vi "Argos_K_4.2 (SUPTNIK Customized Edition).vi"(0 "PID 1 COM":refnum<visa-resource-name>="COM1", 1 "Setpoint\n START":bool, 2 "Write to File":bool, 3 "SP 1 input (°C)":dbl=20.0 min=0.0 max=1300.0, 4 "Intervall (s)":u32=1 max=600, 5 "Write/\nRead":bool=TRUE, 6 "Delay (ms)":u32=500 min=100 max=600000, 7 "Auto Tune":bool, 9 "Standby":bool, 11 "Reset\nSTOPP":bool, 12 "ON":bool=TRUE caption="OFF", 13 "Get Values":bool, 15 "File Path":path) -> (8 "(°C)":dbl format="%#.3f", 14 "SP 1 is (°C)":dbl)   [LabVIEW 2013]
doc: "1. Verwendung\n\nDas Programm dient der Steuerung und Abfrage des Thermocontrollers I3252 und dem Auslesen von zwei VC 840 Messgeräten und einem Druckmessgerät Pfeiffer Single Gauge. \nDie Messgeräte werden Standardmäßig ausgelesen und erst nach Betätigung des Schalters \"Write to File\" in einer Textdatei abgespeichert. Das Eingabefeld \"Intervall\" legt den Abstand der Messpunkte fest.\nDer Setpoint für den Thermocontroller wird erst nach Betätigung des Tasters \"Setpoint START\" übernommen und angesteuert. Er wird ind den EEPROM des Gerätes geschrieben. Die Regelung kann mit Hilfe des Schalters \"Standby\" unterbrochen werden. Durch den Taster \"Reset STOPP\" kann der Setpoint aus dem EEPROM gelöscht werden.\nDie Eingabeflächen \"Constant\" und \"Thickness\" dienen der Berechnung des spezifischen Widerstands.\nDie Eingabeflächen \"User\" und \"Sample\" werden in den Header der Textdatei übernommen.\nDer Indikator \"File Path\" zeigt den aktuellen Speicherort der Textdatei an. Dieser wird nach ausschalten des Schalters \"Write to File\" gelöscht. Bei erneuten Schreiben muss ein neuer Speicherort gewählt werden. Bei Wahl desselben Speicherorts werden sämtliche bereits gespeicherte Daten gelöscht.\n\n\n2. Erläuterungen zum Blockdiagramm\n2.1 äußere Sequenz\nDie äußerte Sequenz besteht aus fünf Frames. Der erste dient der Initialisierung der Ports. Der zweite dient als Verzögerung um dem Programm genug Zeit zu geben die Ports zu öffnen. Jedoch senden die beiden VC 840 bereits Informationen an den Computer die in einem Puffer zwischengespeichert werden. Im dritten Frame wird dieser Puffer geleert. Somit kommt es zu keinem Framing Error. Desweiteren wird in diesem Frame die Startzeit der Messungen genommen. Im vierten Frame wird die eigentliche Messung und Verarbeitung der Daten durchgeführt. Die while-Schleife wird nur durch Auftreten eines Fehlers oder durch Betätigung des Stopbuttons auf dem Front Panel in der oberen linken Ecke unterbrochen. Im fünften und letzten Frame werden die Ports wieder geschlossen und beim Auftreten eines Fehlers wird das Programm automatisch gestoppt. Falls kein Fehler auftritt wird die Sequenz von vorne abgearbeitet.\n\n2.2 while-Schleife und innere Sequenz\n2.2.1 \"Event Structure\"\n2.2.1.1 Allgemein\nDer erste Frame beinhaltet ein \"Event Structure\". Dieser reagiert auf insgesamt elf verschiedene Ereignisse. Falls keines dieser Ereignisse auftreten sollte, warte die Struktur eine Millisekunde bevor die \"Event Structure\" verlassen wird. Die übrigen Ereignisse treten ein, wenn der entsprechende Kontroller eine Werteänderung erfährt.\n\n2.2.1.2 Event: Setpoint\nDieser Case besteht von außen nach innen aus einer Stacked Sequence, einer for-Loop und einer Flat Sequence die wiederum zwei \"Case Structures\" enthält. Als erstes wird bei dem Schalter \"Setpoint START\" der Blinkmodus aktiviert und bei dem Schalter \"Read Temperature\" deaktiviert. Danach folgt das eigentliche setzen des Temperatursollwerts. In der ersten Iteration wird dem Controller I3252 ein Schreibbefehl gesendet. Theoretisch kann der Setpoint in den RAM oder in den EEPROM geschrieben werden. Diese Auswahl erfolgt mit Hilfe des Schalters \"RAM\". Da das Schreiben in den RAM -Speicher aber aus diversen Gründen nicht erwünscht ist, wurde es nicht implementiert. Eine nachträgliche Implementierung ist aber leicht möglich, in dem die untere String-Konstante \"*P012\" durch \"*W012\" ersetzt wird. An diesem Befehl wird eine fünfstellige Hexadezimalzahl angehängt, die den Sollwert wiedergibt. Der Sollwert wird vorher mit zehn multipliziert, da das Komma standardmäßig nach der ersten Ziffer festgesetzt wurde (Bsp.: 800 wird gesendet um 80 einzustellen). Dieser Befehlsstrang wird an das Gerät mittels des SubVIs \"Comm_Interface\", auf welches später noch näher eingegangen wird, weitergegeben. Der durch das Gerät zurückgegebene String wird nicht verarbeitet.\nDie zweite Iteration dient dem Auslesen des eingestellten Sollwertes. Wahlweise kann der RAM- oder der EEPROM-Speicher ausgelesen werden. Die eigentliche Verarbeitung des Ausgabestrings erfolgt durch das SubVI \"Edit Setpoint\".\nDie Implementierung zur Einstellung des zweiten Setpoints erfolgt durch kopieren der ersten beiden Fälle und ersetzen der \"1\" im Befehf durch eine \"2\" (Bsp.: \"*P012\" zu \"*P022\"). Es darf aber nicht vergessen werden, dass dann ebenfalls die Anzahl der Iterationen angepasst werden muss.\nAls letztes wird der Blinkmodus des Schalters \"Setpoint START\" wieder deaktiviert.\n\n2.2.1.3 Event: Standby\nDieses Ereignis aktiviert bzw. deaktiviert als erstes den Blinckmodus des entsprechenden Schalters und sendet danach den Befehl zum aktivieren (\"*D03\") oder zum deaktivieren (\"*E03\") des Standbymodus an den Thermocontroller.\n\n2.2.1.4 Event: Set Command \nDer in das Feld \"Command shall be\" eingegebene Befehl wird an den Thermocontroller übermittlet. Die korrekte Form des Befehls ist im \"Communication Manuel\" nachzuschlagen. Das \"*\"-Zeichen wurde allerdings schon implementiert und muss somit nicht mit eingegeben werden.\n\n2.2.1.5 Event: Reset\nIn der ersten Iteration wird der Reset-Befehl an den Thermocontroller gesendet. In Folge wird der gesamte EEPROM-Speicher gelöscht. Deshalb wird in der zweiten Iteration der Setpoint aktualisiert. Dieser Befehl hat keinen Einfluss auf den RAM-Speicher. Die anschließende Wartezeit ist auf vier Sekunden festgesetzt und wurde empirisch ermittelt. Diese Zeit benötigt das Gerät um den Reset durchzuführen und für die Kommunikation wieder zur Verfügung zu stehen.\n\n2.2.1.6 Event: Auto Tune\nEs ist festgeschrieben, dass der Setpoint für die \"Auto Tune\"-Funktion wenigstens 20°C über der aktuellen Temperatur liegt. Deshalb wird zunächst der aktuelle Temperaturwert ausgelesen. Im zweiten Schritt werden zu diesem Wert zwanzig addiert und der Setpoint wird in den RAM-Speicher geschrieben. Das Schreiben in diesen Speicher ist nötig, da die \"Auto Tune\"-Funktion\" erst nach einem Reset startet. Im dritten Schritt wird der eigentliche Befehl für den \"Auto Tune\" gesendet (siehe dazu \"Communication Manuel\" S.27). Als vierte und letzte Iteration der for-Schleife folgt der bereits erwähnte Reset-Befehl. Der Temperatursollwert, der im RAM-Speicher eingetragen ist, muss zum Schluss wieder auf 0°C gesetzt werden. Die Zeit für die Ausführung des \"Auto Tune\"-Befehls wurde empirisch ermittelt und 45 s festgesetzt.\n\n2.2.1.7 Event: Write LOW/HI\nDieses Ereignis setzt die am Analogausgang anliegende Spannung fest. Normalerweise beträgt dieser Spannungswert 0-10 V. Das angeschlossene Netzteil verträgt aber maximal nur 2,3 V. Aus diesem Grund wird der \"%HIGH\" auf 23 gesetzt. Somit beträgt die maximal anliegende Spannung nur noch 23% von der maximal möglichen, d.h 2,3V. Ein niedrigerer Wert ist jederzeit möglich, genauso wie ein höherer für den Parameter \"%LOW\". Diese werden zunächst nacheinander in den RAM-Speicher geschrieben und anschließend wieder ausgelesen.\n\n2.2.1.8 Event: Set PID\nDie Werte für den PID-Regler können sowohl mit Hilfe der \"Auto Tune\"-Funktion, als auch manuell eingestellt werden. Es wird wiederum zwischen dem Schreiben in den RAM- und dem EEPROM-Speicher unterschieden. Zunächst werden die Werte für \"P\", \"I\" und \"D\", in dieser Reihenfolge, gesetzt und danach die aktuellen Werte ausgelesen.\n\n2.2.1.9 Event: Get Values\nDieses Ereignis hat zur Folge, dass die Werte für \"P\", \"I\", \"D\", \"%LOW\", \"%HIGH\" und des Setpoints wahlweise aus dem RAM- oder EEPROM-Speicher gelesen werden. Die aktuellen Werte werden nicht nur in die entsprechenden Anzeigefelder übernommen, sondern auch in die entsprechenden Eingabefelder, mit Ausnahme des Temperatursollwerts. \n\n2.2.1.10 Event: RAM\nPrinzipiell kann zwischen dem Schreiben in den RAM- oder EEPROM-Speicher des Thermocontrollers gewählt werden. Die entsprechende Schalterposition auf dem Frontpanel zeigt den aktuell verwendeten Speicher an. Die Anzeigewerte werden bei jedem Umschalten aktualisiert und sind im entsprechenden Speicher eingetragen. Die Implementierung ist identisch mit der des Ereignisses \"Get Values\". Es gilt zu beachten, dass die Werte für \"%LOW\" und \"%HIGH\" nur in den RAM-Speicher geschrieben werden können und somit auch nur aus diesem ausgelesen werden können.\n\n2.2.1.11 Event: Set Gauge to Zero\nMit Hilfe der SubVIs \"Get Pressure\" und \"Offset Display\" werden die Werte für den alten und den neuen Offset und der durch den zweiten Drucksensor ermittelt Druck ermittelt. \n\n2.2.1.12 Event: Write to File\nSollte der Schalter \"Write to File\" aktiviert werden, d.h. Schalterposition oben, so wird zunächst durch das SubVI \"Header\" ein Header für die unter \"File Path\" definierte Datei angelegt. Alle Werte, die bereits in der entsprechenden Datei stehen, werden dabei gelöscht.\n\n2.2.2 \"Timed Structures\"\nIm dritten Frame der inneren Sequenz werden die Werte für Zeitpunkt, Temperatur, Spannung, Strom und Druck ermittelt. Damit die Werte zum gleichen Zeitpunkt aufgenommen werden, werden \"Timed Sequences\" eingesetzt. Mit dem entsprechenden Schalter auf dem Front Panel unter dem Tab \"Settings\" kann gewählt werden, ob das entsprechende Gerät ausgelesen werden soll oder nicht. Die einzelnen Sequenzen werden parallel abgearbeitet, womit die Prozesszeit von diesem Frame durch der zeitintensivsten Sequenz abhängt. Dies ist in aller Regel das Auslesen der Temperatur, da ein \"Delay\" von 500 ms oder größer benötigt wird, um den Controller ordentlich ansprechen zu können.\nDie Systemzeit wird durch das SubVI \"System Time in Seconds\" in Sekunden umgerechnet und der in dem Parameter \"Starttime\" gespeicherte Wert wird abgezogen. Somit werden die Sekunden seit dem Start des Programms gezählt.\n\n2.2.3 restlichen Frames\nIm zweiten Frame wird das Intervall zwischen den einzelnen Messwerten festgelegt. Dabei wird der Wert des Parameters \"Delay\" abgezogen. Dieser Wert beträgt im Normalfall 500 ms und ist somit nicht vernachlääsigbar.\nDer Vierte Frame beinhaltet die Umrechnung des Temperatur-Strings in einen Temperaturwert durch das SubVI \"Edit Tmperature\", die Berechnung des spezifischen Widerstands durch das SubVI \"Resistivity Calculation\" und die Überprüfung des Druckwerts. Auch werden die neu gewonnen Werte in das entsprechende Shift-Register übernommen. Falls der Druckwert einen in dem Parameter \"Pressure Limit (mbar)\" festgelegten Grenzwert überschreiten sollte, wird der Thermocontroller automatisch in den Standby-Modus versetzt. Des Weiteren wird der Schalter \"Standby\" solange gesperrt, wie der Druck oberhalb des Grenzwertes liegt. Wenn der Druck wieder unter den Grenzwert gesunken ist, wird der Standby-Befehl nicht automatisch aufgehoben, sondern muss vom Benutzer durch Betätigung des entsprechenden Schalters gegeben werden.\nIm fünften Frame werden die Diagramme erstellt. Dabei wird jedes Mal von neuem das gesamte Shift-Register als Graph dargestellt. Weiterhin werden die Messwerte in ein 1D-Array geschrieben.\nDer sechste und letzte Frame beinhaltet den eigentlich Schreibvorgang der Messwerte in eine Textdatei und die Überprüfung ob ein Fehler vorliegt.\n\n2.3 SubVIs\n2.3.1 Allgemein\nDie SubVIs für die Messgeräte VC840 und das Druckmessgerät wurden aus anderen Quellen übernommen. \n\n2.3.2 \"Header\"\nIn den Header wird zunächst das aktuelle Datum und die aktuelle Zeit übernommen. Die ausgewählte Datei wird dabei überschrieben. Danach wird der Name des Benutzers und der Probe übernommen. Zum Schluss werden die Einheiten in einer Reihe, durch einen Tabulator getrennt, in den Header geschrieben.\n\n2.3.3 \"I3252 Comm Interface\"\nDieses VI stellt die Kommunikation mit dem Thermocontroller her und gibt den Ausgabe-String zurück.\n\n2.3.4 \"I3252 Edit Setpoint\"\nIm Ausgabe-String vom Thermocontroller ist an der vierten Stelle die Stelle des Dezimalpunktes verschlüsselt. Dieses Hexadezimalzahl wird herausgefiltert und an ein \"ENUM Controller\" übergeben. Dieser weist der Hexadezimalzahl eine Nummer zu, mit welcher ein Wert aus einem Array entnommen wird. Dieser Wert dient als Quotient. Der tatsächliche Wert kann somit errechnet werden.\n\n2.3.5 \"I3252 Edit Temperature\"\nDer Temperatur-String, der vom Thermocontroller zurückgegeben wird, wird in eine Dezimalzahl umgewandelt. Manchmal kommt es aus zu Dropouts, die durch dieses Programm herausgefiltert werden. Der letzte Wert wird dabei in einer \"Feedback Node\" gehalten unter der Annahme, dass sich der Temperaturwert nicht sprunghaft ändert.\n\n2.3.6 \"Resistivity Calculation\"\nDer spezifische Widerstand wird nach folgender Formel ausgerechnet. Dabei entspricht t der Dicke der Probe und C ist eine Konstante.\nrho=C*pi*t*U/(ln( 2)*I)\n\n2.3.7 \"System Time in Seconds\"\nZunächst wird die aktuelle Systemzeit ausgelesen. Danach wird diese in Stunden, Minuten und Sekunden aufgeteilt, alles in Sekunden umgerechnet und letztendlich addiert."
uses:
  <vilib>/Platform/TimedLoop/XDataNode/timing_clust.ctl
  <vilib>/Platform/TimedLoop/XDataNode/nitl_modes.ctl
  <vilib>/Platform/TimedLoop/XDataNode/wakeup.ctl
  <vilib>/Instr/_visa.llb/VISA Configure Serial Port (Instr).vi
  <vilib>/Platform/TimedLoop/scheduler/LVUserAPI/_suppVIs/Create_1kHz_TSource.vi
  <vilib>/Utility/file.llb/Write To Spreadsheet File (DBL).vi
  <vilib>/Platform/TimedLoop/XDataNode/XDataNode.xnode
  <vilib>/Platform/TimedLoop/XDataNode/XDNodeRunTimeDep.lvlib
  Argos0v7/Dependencies/Pfeiffer TPG261+262 Single+Dual Gauge/Dual Gauge.lvlib
panel:
  out "appended array":dbl[](array[numeric])
  in  "Tab Control":T1(tab)
  in  "Sample":string
  in  "User":string
  out "Thermocouple (Sample holder 1)":cluster{dbl[], dbl[]}(graph)
  out "current time (s)":dbl
  out "data logger intervall (s)":dbl
  out "loop time (s)":dbl
  in  "stop":bool
  out "TPG 1":cluster{dbl[], dbl[]}[](graph)
  out "Pressure Baratron 2":dbl format="%#_4e"
  out "Pressure FullRange 2":dbl format="%#_3e"
  out "Pyrometer Temperature °C":cluster{dbl[], dbl[]}(graph)
  out "Pyro Temp":dbl format="%.2f"
  out "Pressure OpenPort":cluster{dbl[], dbl[]}(graph)
  out "Pressure OpenPort2":dbl caption="current"
  in  "Emissivity\n(eg: 0500)":string
  in  "Pyro COM Port":refnum<visa-resource-name>="COM3"
  in  "Pyrometer":bool caption="ON\nOFF"
  out "status 2":bool caption="Status"
  out "code 2":i32 caption="Code"
  in  "ON (TPG 2)":bool caption="OFF"
  in  "TPG 2 COM":refnum<visa-resource-name>="COM8"
  out "Pressure Gauge 2#2":dbl format="%.3e"
  out "Pressure Gauge 2#1":dbl format="%.3e"
  out "Status Gauge 2#2":i32(ring) items=["data OK", "underrange", "overrange", "sensor error", "sensor off", "no sensor", "ID error"]
  out "Status Gauge 2#1":i32(ring) items=["data OK", "underrange", "overrange", "sensor error", "sensor off", "no sensor", "ID error"]
  out "code":i32 caption="Code"
  out "status":bool caption="Status"
  in  "Set Gauge to Zero":bool
  out "Status Gauge 1#2":i32(ring) items=["data OK", "underrange", "overrange", "sensor error", "sensor off", "no sensor", "ID error"]
  out "Pressure Gauge 1#2":dbl format="%.3e"
  out "Pressure Gauge 1#1":dbl format="%.3e"
  out "Status Gauge 1#1":i32(ring) items=["data OK", "underrange", "overrange", "sensor error", "sensor off", "no sensor", "ID error"]
  in  "TPG 1 COM":refnum<visa-resource-name>="COM5"
  in  "Pressure Limit (mbar)":dbl=1.0 min=0.0 max=1100.0
  out "Current Offset (mbar)":dbl
  in  "ON (TPG 1)":bool=TRUE caption="OFF"
  in  "ON":bool caption="OFF"
  in  "VC 840 2":refnum<visa-resource-name>="COM8"
  out "Reading 2":dbl format="%_4f"
  out "Mode 2":enum16{"?", "Diode", "Beep", "DC", "AC"}(ring)
  out "Unit 2":string
  in  "VC 840 1":refnum<visa-resource-name>="COM8"
  out "Reading 1":dbl format="%_4f"
  out "Mode 1":enum16{"?", "Diode", "Beep", "DC", "AC"}(ring)
  out "Unit 1":string
  out "Status 1":T2
  out "Status 2":T2
  in  "ON":bool caption="OFF"
  out "% HIGH Istwert":u32
  out "% LOW Istwert":u32
  in  "% High Sollwert":u32=23 max=24
  in  "% LOW Sollwert":u32 max=25
  in  "RAM":bool=TRUE caption="EEPROM"
  out "D (Rate) IstWert":u32
  out "I ( Reset1) Istwert":u32
  out "P (PB1) Istwert":u32 caption="actual value"
  in  "D (Rate) Sollwert":u32 max=3999
  in  "I ( Reset1) Sollwert":u32 max=3999
  in  "P (PB1) Sollwert":u32 caption="set value" max=9999
  in  "Set Command":bool
  in  "Set PID":bool
  in  "Write LOW/HI":bool
  in  "Flow Control":u16(ring) items=["None"=0, "XON/XOFF"=1, "RTS/CTS"=2, "DTR/DSR"=4]
  in  "Stop Bits":u16(ring)=10 items=["1.0"=10, "1.5"=15, "2.0"=20]
  in  "Parity":u16(ring)=1 items=["None", "Odd", "Even", "Mark", "Space"]
  in  "Data Bits":u16=7 min=5 max=8 step=1
  in  "Baud Rate":u32=9600
  out "Command output":string
  in  "Command input":string
  out "Get Actual Set Point":dbl
  in  "Get SetPoint":bool
  in  "Setpoint":dbl=10.0
  in  "Minutes":dbl
  in  "Hours":dbl
  in  "Soak Minutes":dbl=1.0
  in  "Soak Hours":dbl
  in  "Ramp":bool
  out "Current":cluster{dbl[], dbl[]}(graph)
  out "Voltage":cluster{dbl[], dbl[]}(graph)
  out "Voltage (V)":dbl format="%.4e"
  out "Current (A)":dbl format="%.4e"
  out "Resistivity":cluster{dbl[], dbl[]}(graph)
  out "Resistivity (Ohm*cm)":dbl format="%.3e"
  out "Pirani (VVP1 Scroll)":cluster{dbl[], dbl[]}(graph)
  in  "4PP constant":dbl min=0.0 max=5.0
  in  "Thickness (nm)":dbl min=0.0
  out "Pressure Pirani 2":dbl format="%#_3e"
  # "set \nvalue"
  # "actual \nvalue"
  # "T (°C)"
  # "mbar"
  # "mbar"
  # "mbar"
  # "Pressure Measurement \n(Pfeiffer TPG261)"
  # "Pyrometer"
  # "limit (mbar)"
  # "Multimeter\n#1 (VC 840)"
  # "Multimeter\n#2 (VC 840)"
  # "PID Controller (Omega Newport i3252)"
  # "P"
  # "I"
  # "D"
  # "% Low"
  # "% High"
  # "Ramp And Soak Toolkit"
  # "Ramp"
  # "Soak"
  # "mbar"
  # "Authors:  Daniel Schuster (sir-dan@web.de)\n                 Steffen Cornelius (s.cornelius@hzdr.de)\n                 Nico Spahn (x)\n\n                 premade SubVIs for readout of Pfeiffer gauge and VC840 Multimeters were used\n                 SubVI \"I3252_Comm_Interface\" is based on a modified Labview example\n\nRelease:  v1.0    \n\nVersion History:\n\nv1.1  -    28.06.2011\n             - Format des Files geändert von %.3f auf %g\n             - maximale Eingabewerte für PID begrenzt\nv1.2  -    12.07.2011\n             - Anzeige p,rho, U, V auf Scientific geändert\n             - y-Achse p,rho auf Log geändert\n             - numerische Zeitanzeige hinzugefügt\n             - 4PP Constant: pi/ln(2)=4,532 set as the default value\nv1.3  -    25.07.2011\n             - Zeitvariable auf EXT geändert, um Sprünge in Diagrammen loszuwerden\nv1.4  -   27.07.2011\n             - ALLE Variablen auf DBL zurückgesetzt wegen Formatierungsproblem im File\n             - Zeitberechnung neu gemacht (Tick count differenzen) -> Zeitsprünge korrigiert ?\n             - Delay/Intervall überarbeitet\nv1.5  -   05.12.2012\n                - Austausch der alten Pfeifer SubvIs durch neue -> nun alle 4 Kanäle des DualGauge\n                                                                                                         Controllers gleichzeitig auslesbar\n                - neue Pfeiffer SubVIs verwendet in Druckwertauslesung und Offset Berechnung des Baratron\n                  Druckes (COM5 Sensor1)\n                - Neuarragement des GUI -> FullRange und Baratron neben Temperatur auf Haupseite zu sehen\n                                                                   Pirani und OpenPort auf Meas.2 zu sehen\n                                                                   Diagnose Seite umfasst nun auch Widerstandsdiagramm\n                - Änderungen der Settingseite -> nun alle 4 Drucksensoren mit aktuellem Messwert und Gerätestatus\n                                                                           zu sehen\n                - The readout of the PID-Temperature Controller and the VC840 Multimeters was not modified\nv1.73  -  18.10.2013\n                - Layout Änderungen\nv.1.8   -  19.01.2014\n                - Änderung Layout Settings Tab\n                - Trennung der beiden TPG Dual Gauge Controls\n                -"
  # "Version 1.73    - last change 18.10.2013"
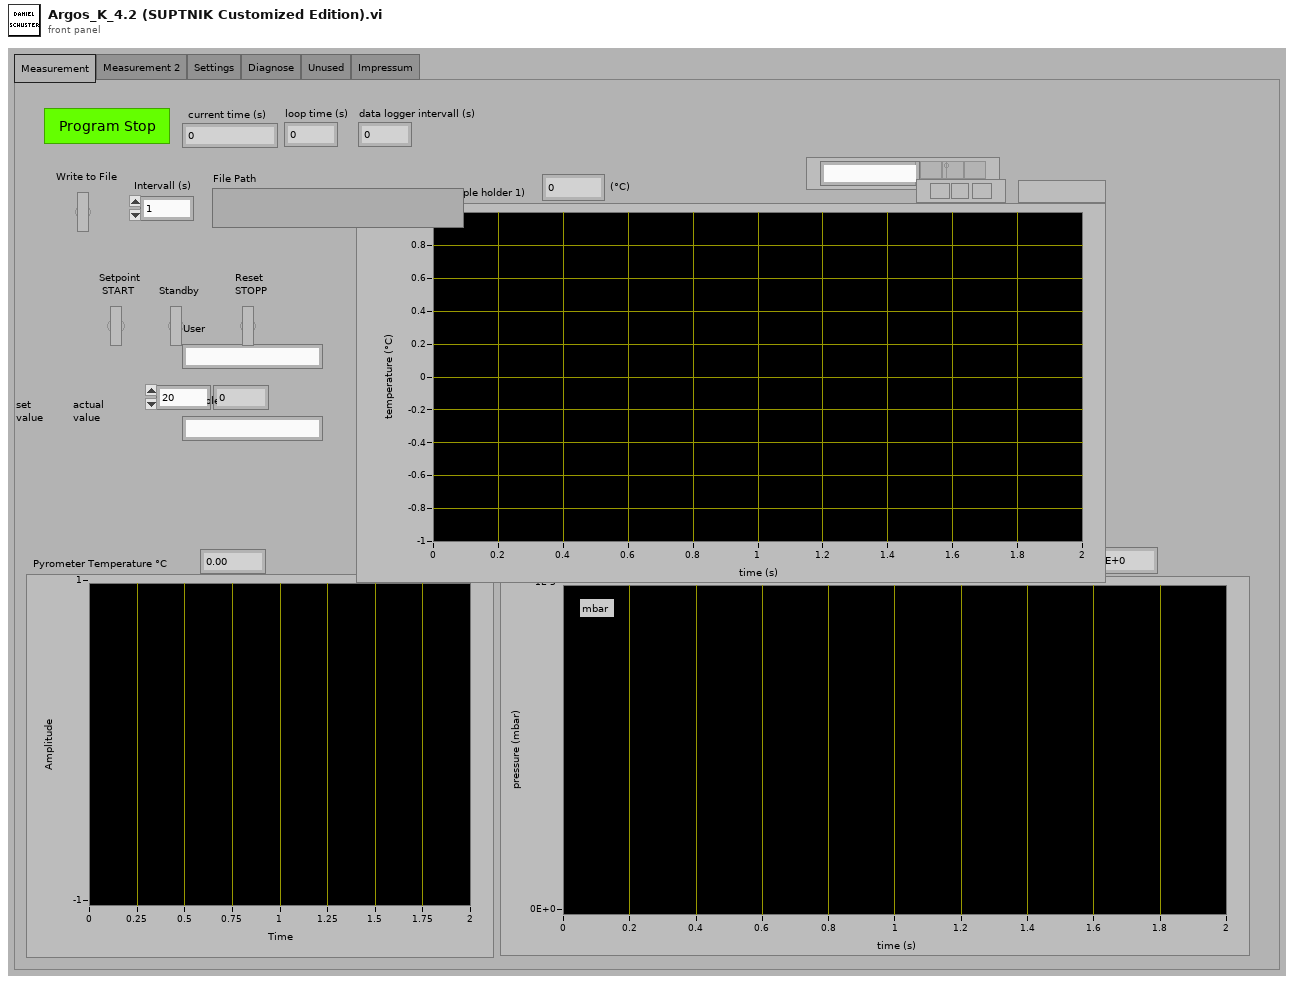
[diagram p1: front panel]
types:
  T1 = enum32{"Measurement", "Measurement 2", "Settings", "Diagnose", "Unused", "Impressum"}
  T2 = cluster{"Low Bat":bool, "Auto":bool, "Delta":bool, "Hold":bool, "RS232":bool}
  T3 = typedef "XDNodeRunTimeDep.lvlib/timing_clust.ctl" = cluster{"Expected End [f-1]":u64, "Actual End [f-1]":u64, "Finished Late? [f-1]":bool, "Expected End [i-1]":u64, "Actual End [i-1]":u64, "Finished Late? [i-1]":bool, "Expected Start [i]":u64, "Actual Start [i]":u64, "Expected Start [f]":u64, "Actual Start [f]":u64, "Source Name":string, "Structure Name":string, "Period":i64, "Deadline":i64, "Offset":i64, "Start":i64, "Priority":i32, "Timeout":i32, "Mode":T4, "Wakeup Reason":T5, "Error":errorcluster, "Source Type":string, "Secondary Source Type":string, "Global End Time":u64, "Global Start Time":u64, "Frame Duration":u64, "Iteration Duration":u64, "Assigned CPU":i32, "I/O Scan Engine Mode":u32}
  T4 = typedef "XDNodeRunTimeDep.lvlib/nitl_modes.ctl" = enum32{"No Change", "Process missed periods, maintain original phase", "Discard missed periods, maintain original phase", "Process missed periods, ignore original phase", "Discard missed periods, ignore original phase"}
  T5 = typedef "XDNodeRunTimeDep.lvlib/wakeup.ctl" = enum32{"Normal", "Aborted", "Asynchronous wakeup", "Timing source error", "Timed loop error", "Timeout"}
  T6 = enum8{"Enabled", "Disabled", "Disabled and Grayed Out"}
  T7 = cluster{"VISA resource name out":refnum<visa-resource-name>, "error out":errorcluster, "Delay (ms)":u32, "Write/\nRead":bool}
  T8 = cluster{"TPG 2 COM":refnum<visa-resource-name>, "error out":errorcluster}
  T9 = cluster{"COM out":refnum<visa-resource-name>, "Cluster (Ausgang)":errorcluster}
  T10 = cluster{"Pressure Gauge#1":dbl, "Pressure Gauge#2":dbl}
  T11 = cluster{"TPG 1 COM":refnum<visa-resource-name>, "error out":errorcluster}
  T12 = cluster{"COM out":refnum<visa-resource-name>, "error out":errorcluster, "COM out":refnum<visa-resource-name>, "error out":errorcluster}
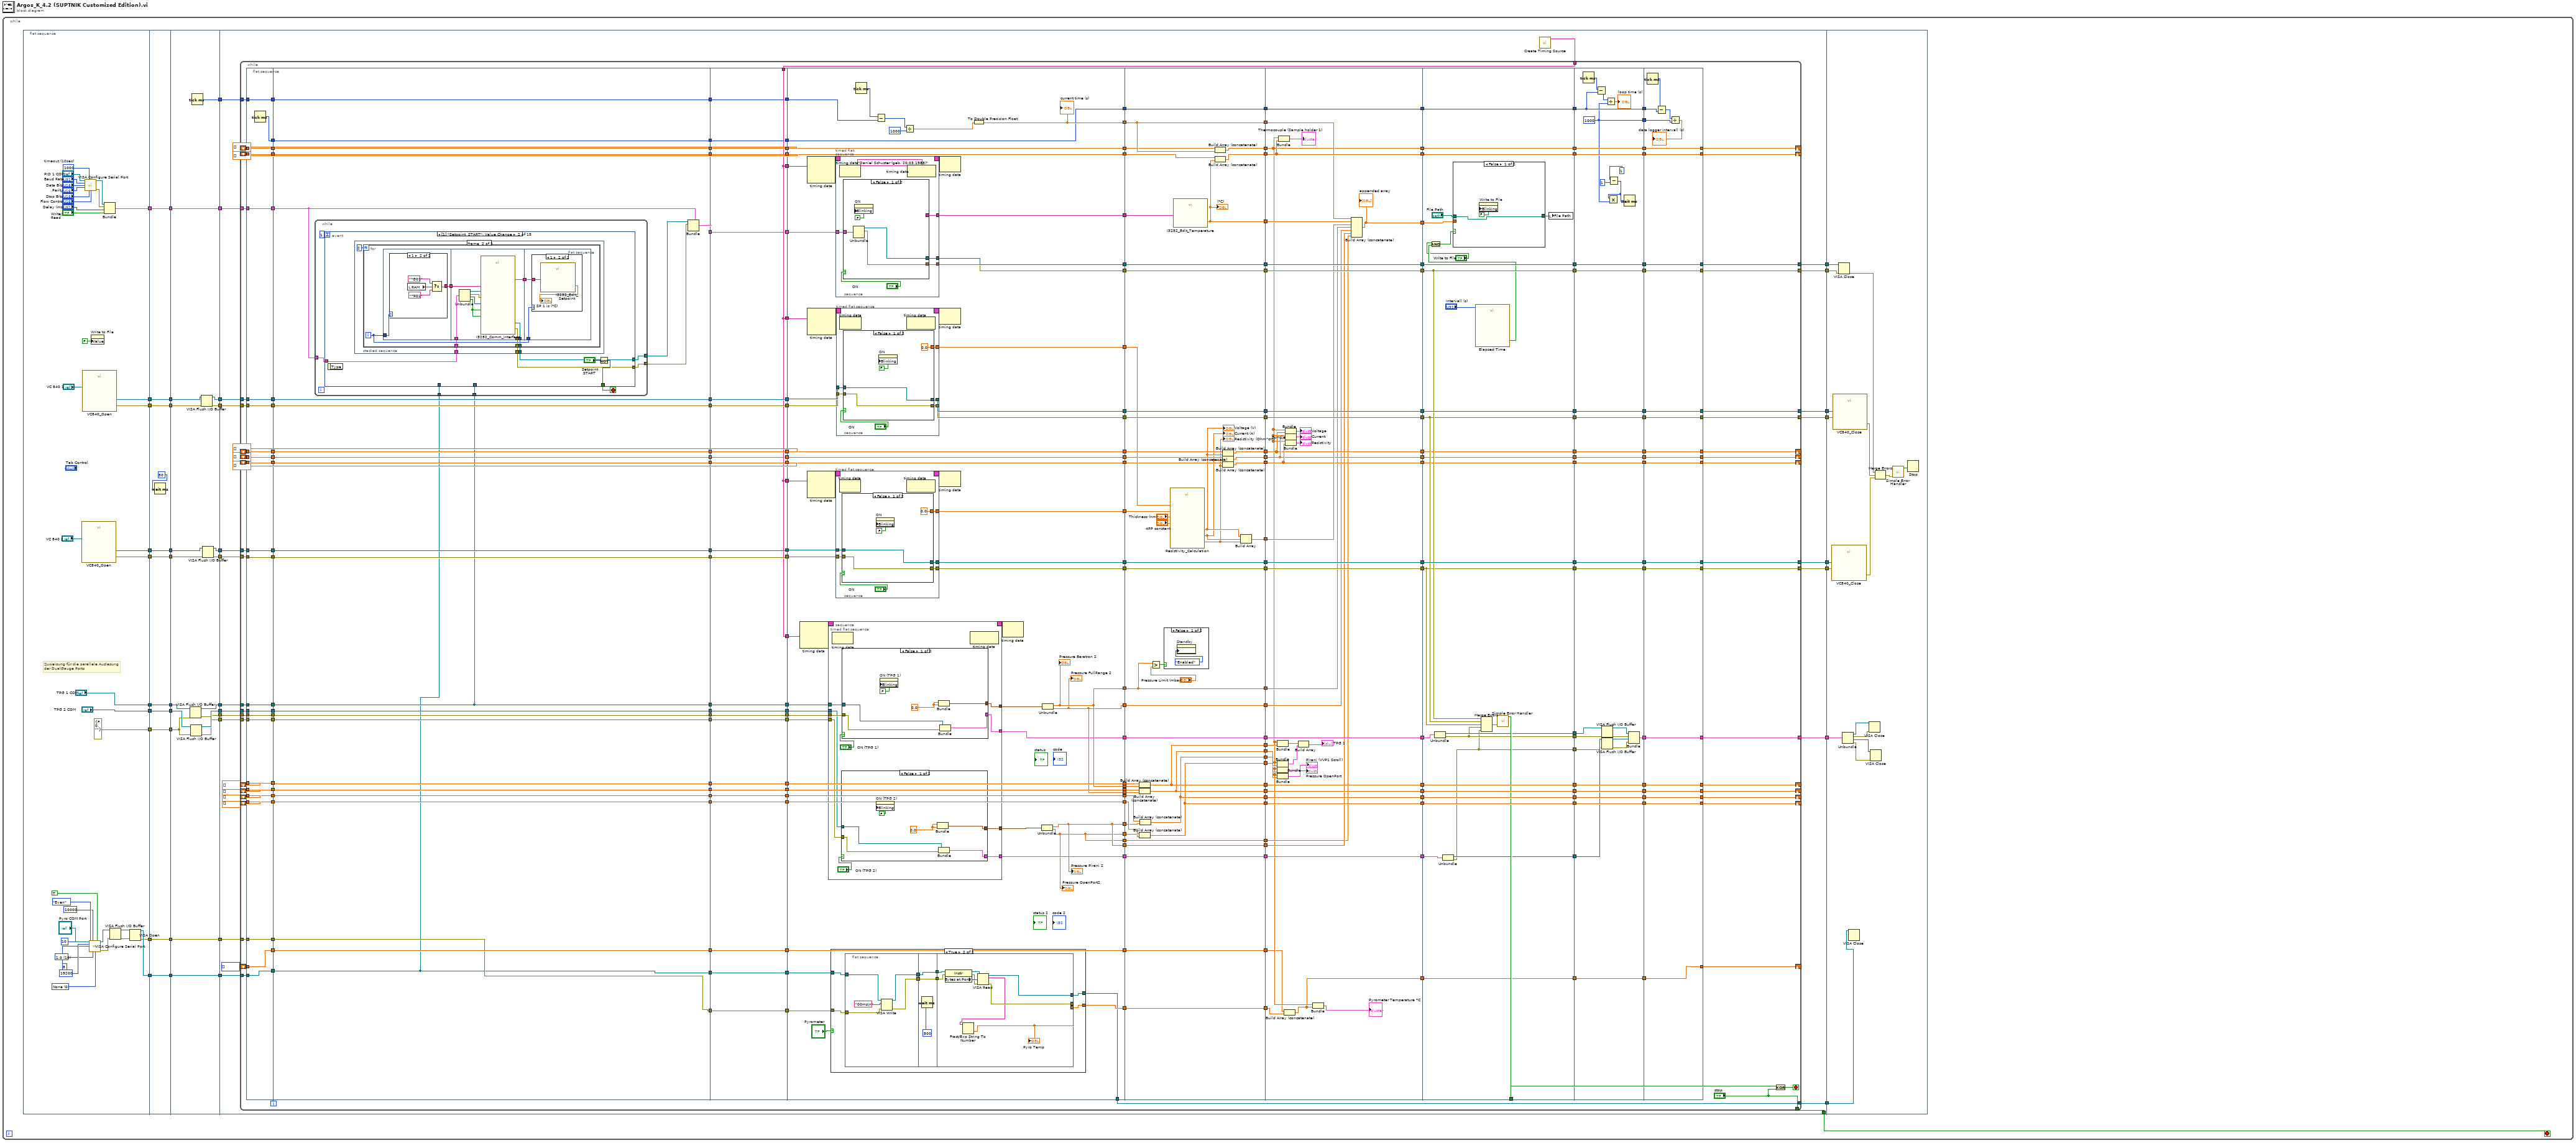
[diagram p0: block diagram]
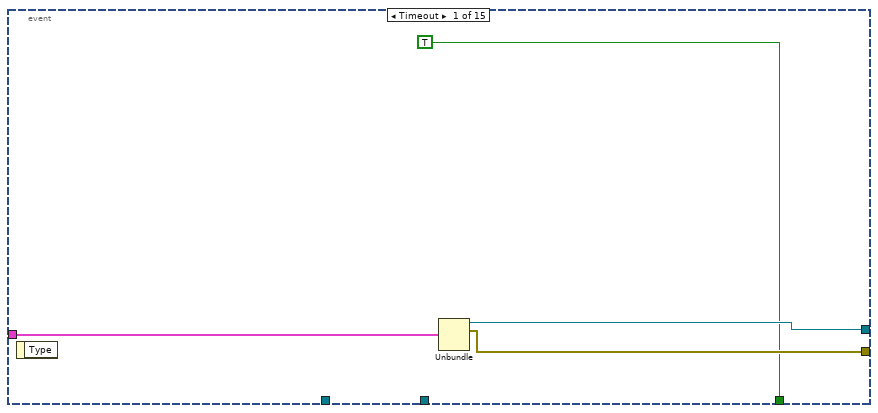
[diagram p2: hidden frame]
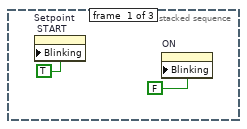
[diagram p3: hidden frame]
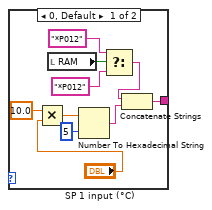
[diagram p4: hidden frame]
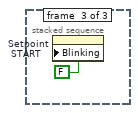
[diagram p6: hidden frame]
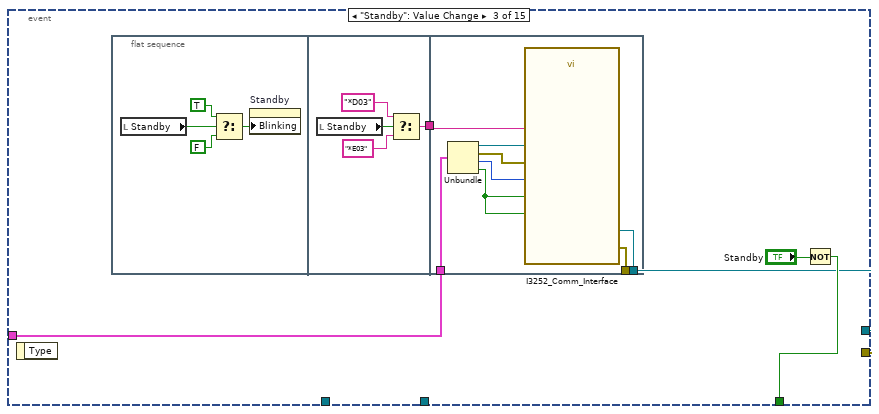
[diagram p7: hidden frame]
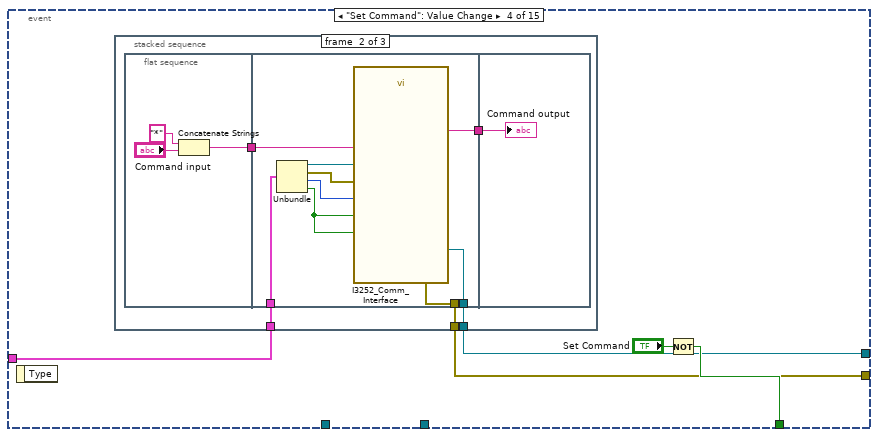
[diagram p8: hidden frame]
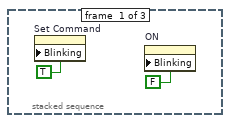
[diagram p9: hidden frame]
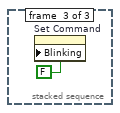
[diagram p10: hidden frame]
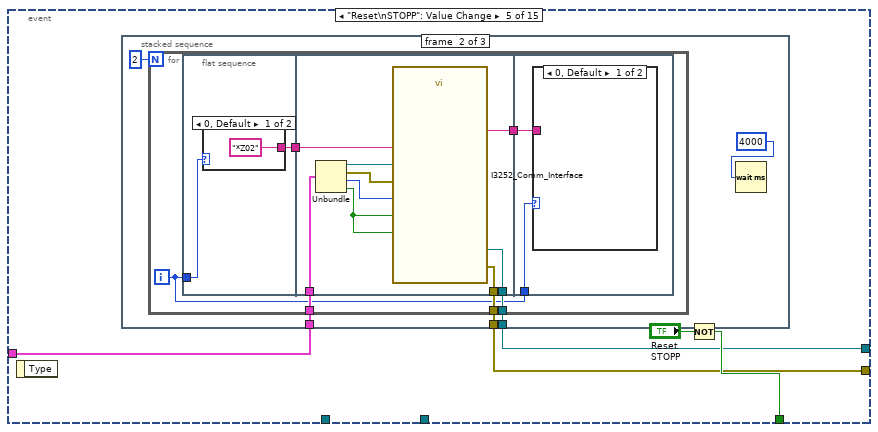
[diagram p11: hidden frame]
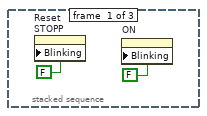
[diagram p12: hidden frame]
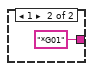
[diagram p13: hidden frame]
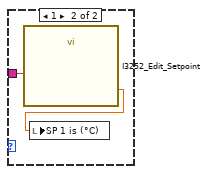
[diagram p14: hidden frame]
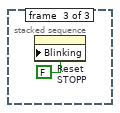
[diagram p15: hidden frame]
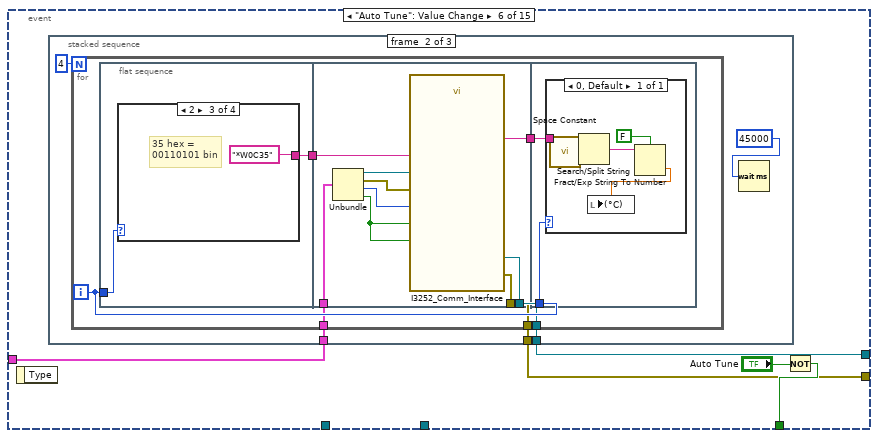
[diagram p16: hidden frame]
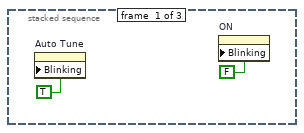
[diagram p17: hidden frame]
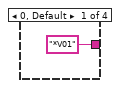
[diagram p18: hidden frame]
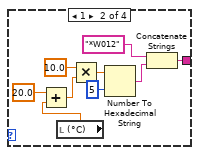
[diagram p19: hidden frame]
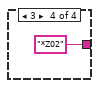
[diagram p20: hidden frame]
diagram:
  n1 = while {
    stop <- w13 stop-if-true
    n2 = flat-sequence {
      tunnel: [w77] -> w41
      tunnel: [w78] -> w40
      tunnel: [w63] -> w39
      tunnel: [w76] -> w38
      tunnel: [w75] -> w37
      tunnel: ["TPG 1 COM"] -> w36
      tunnel: ["TPG 2 COM"] -> w35
      tunnel: [errorcluster {"status"=FALSE, "code"=0, "source"=""} ("Fehler (Eingang)")] -> w10
      tunnel: [w43] -> w7
      tunnel: [w42] -> w2
      tunnel: w41 -> [w89]
      tunnel: [w89] -> w34
      tunnel: w40 -> [w88]
      tunnel: [w88] -> w33
      tunnel: w39 -> [w87]
      tunnel: [w87] -> w32
      tunnel: w38 -> [w86]
      tunnel: [w86] -> w31
      tunnel: w37 -> [w85]
      tunnel: [w85] -> w30
      tunnel: [w83] -> w29
      tunnel: w36 -> [w83]
      tunnel: [w82] -> w28
      tunnel: w35 -> [w82]
      tunnel: [w81] -> w11
      tunnel: w10 -> [w81]
      tunnel: w7 -> [w80]
      tunnel: [w80] -> w6
      tunnel: [w79] -> w3
      tunnel: w2 -> [w79]
      tunnel: w34 -> [w102]
      tunnel: [w101] -> w27
      tunnel: w33 -> [w103]
      tunnel: [w100] -> w26
      tunnel: w32 -> [w108]
      tunnel: [w108] -> w25
      tunnel: w31 -> [w105]
      tunnel: [w106] -> w24
      tunnel: w30 -> [w104]
      tunnel: [w107] -> w23
      tunnel: [w99] -> w22
      tunnel: [w97] -> w21
      tunnel: w29 -> [w98]
      tunnel: [w96] -> w20
      tunnel: w28 -> [w95]
      tunnel: w11 -> [w94]
      tunnel: [w93] -> w9
      tunnel: [w92] -> w8
      tunnel: w6 -> [w91]
      tunnel: [w91] -> w5
      tunnel: [w90] -> w4
      tunnel: w3 -> [w90]
      tunnel: w27 -> [w140]
      tunnel: w26 -> [w139]
      tunnel: w25 -> [w138]
      tunnel: w24 -> [w136]
      tunnel: w23 -> [w135]
      tunnel: [w134] -> w19
      tunnel: [w133] -> w18
      tunnel: [w132] -> w17
      tunnel: [w131] -> w16
      tunnel: [w130] -> w15
      tunnel: [w129] -> w14
      tunnel: w22 -> [w123]
      tunnel: w21 -> [w122]
      tunnel: w20 -> [w121]
      tunnel: [w116] -> w13
      tunnel: [w115] -> w12
      tunnel: w9 -> [w114]
      tunnel: w8 -> [w113]
      tunnel: w5 -> [w111]
      tunnel: w4 -> [w110]
      tunnel: [w109] -> w1
      tunnel: w19 -> [w1512]
      tunnel: w18 -> [w1511]
      tunnel: w17 -> [w1514]
      tunnel: w16 -> [w1513]
      tunnel: w15 -> [w1516]
      tunnel: w14 -> [w1515]
      tunnel: w12 -> [w1509]
      tunnel: w1 -> [w1504]
      frame #0 {
        w50 = u16 10 items=["1.0"=10, "1.5"=15, "2.0"=20] ("stop bits (10: 1 bit)")
        w49 = u16 0 items=["None", "XON/XOFF", "RTS/CTS", "XON/XOFF & RTS/CTS", "DTR/DSR", "XON/XOFF & DTR/DSR"] ("flow control (0:none)")
        w64 = u32 1000  # timeout (10sec)
        # "Zuweisung für die parallele Auslesung\nder DualGauge Ports"
        n3 = call "VC840_Open.vi"("VISA resource name"="VC 840 2") -> ("error out"=w75:errorcluster, "VISA resource name out"=w76:refnum<visa-resource-name>)  [unwired: 1 in, 8 out]
        n4 = call "VC840_Open.vi"("VISA resource name"="VC 840 1") -> ("error out"=w78:errorcluster, "VISA resource name out"=w77:refnum<visa-resource-name>)  [unwired: 1 in, 8 out]
        n5 = call-poly "VISA Configure Serial Port"("VISA resource name"="PID 1 COM", "timeout (10sec)"=w64, "baud rate (9600)"="Baud Rate", "data bits (8)"="Data Bits", "parity (0:none)"="Parity", "stop bits (10: 1 bit)"="Stop Bits", "flow control (0:none)"="Flow Control") -> ("VISA resource name out"=w73:refnum<visa-resource-name>, "error out"=w74:errorcluster)  [unwired: 2 in, 5 out]
        n6 = call-poly "VISA Configure Serial Port"("VISA resource name"="Pyro COM Port", "timeout (10sec)"=u32 10000, "termination char\n(0xA = '\\n' = LF)"=u8 10 ("termination char\n(0xA = '\\n' = LF)"), "Enable Termination\nChar (T)"=TRUE ("Enable Termination\nChar (T)"), "baud rate (9600)"=u32 19200, "data bits (8)"=u16 8, "parity (0:none)"=enum16{"None", "Odd", "Even", "Mark", "Space"}."Even", "stop bits (10: 1 bit)"=w50, "flow control (0:none)"=w49) -> ("VISA resource name out"=w55:refnum<visa-resource-name>, "error out"=w45:errorcluster)  [unwired: 5 in]
        n7 = property on="Write to File" class="Bool (strict)"("Value"=FALSE ("Write to File")) -> ()  [unwired: 2 in, 2 out]
        n8 = Bundle("VISA resource name out"=w73, "error out"=w74, "Delay (ms)"="Delay (ms)", "Write/\nRead"="Write/\nRead") -> (w63:T7)  [unwired: 1 in]
        n9 = VISA Flush I/O Buffer(VISA resource name=w55, error in (no error)=w45) -> (VISA resource name out=w56:refnum<visa-resource-name>, error out=w44:errorcluster)  [unwired: 1 in]
        n10 = VISA Open(error in (no error)=w44, VISA resource name=w56) -> (VISA resource name=w43:refnum<visa-resource-name>, error out=w42:errorcluster)  [unwired: 3 in]
      }
      frame #1 {
        n11 = Wait (ms)(milliseconds to wait=u32 50) -> ()  [unwired: 1 out]
      }
      frame #2 {
        n12 = VISA Flush I/O Buffer(VISA resource name=w98, error in (no error)=w94) -> (VISA resource name out=w97:refnum<visa-resource-name>, error out=w93:errorcluster)  [unwired: 1 in]
        n13 = VISA Flush I/O Buffer(VISA resource name=w95, error in (no error)=w94) -> (VISA resource name out=w96:refnum<visa-resource-name>, error out=w92:errorcluster)  [unwired: 1 in]
        n14 = Tick Count (ms)() -> (millisecond timer value=w99:u32)
        n15 = VISA Flush I/O Buffer(VISA resource name=w102, error in (no error)=w103) -> (VISA resource name out=w101:refnum<visa-resource-name>, error out=w100:errorcluster)  [unwired: 1 in]
        n16 = VISA Flush I/O Buffer(VISA resource name=w105, error in (no error)=w104) -> (VISA resource name out=w106:refnum<visa-resource-name>, error out=w107:errorcluster)  [unwired: 1 in]
      }
      frame #3 {
        n17 = call-poly <vilib>:"Create Timing Source.vi"() -> ("name (out)"=w137:string)  [unwired: 10 in, 1 out]
        n18 = while {
          tunnel: w140 -> [w380]
          tunnel: w139 -> [w379]
          tunnel: w138 -> [w378]
          tunnel: w137 -> [w371]
          tunnel: w136 -> [w364]
          tunnel: w135 -> [w363]
          tunnel: [w359] -> w134
          tunnel: [w358] -> w133
          tunnel: [w356] -> w132
          tunnel: [w354] -> w131
          tunnel: [w352] -> w130
          tunnel: [w350] -> w129
          shift-right: [w323] -> _
          shift-left: dbl[] [] -> [w328]
          shift-right: [w301] -> _
          shift-left: dbl[] [] -> [w336]
          shift-right: [w325] -> _
          shift-left: dbl[] [] -> [w332]
          shift-right: [w298] -> _
          shift-left: dbl[] [] -> [w335]
          shift-right: [w295] -> _
          shift-left: dbl[] [] -> [w334]
          tunnel: w123 -> [w289]
          tunnel: w122 -> [w245]
          tunnel: w121 -> [w241]
          shift-right: [w199] -> _
          shift-left: dbl[] [] -> [w229]
          shift-right: [w197] -> _
          shift-left: dbl[] [] -> [w227]
          shift-right: [w195] -> _
          shift-left: dbl[] [] -> [w225]
          shift-right: [w193] -> _
          shift-left: dbl[] [] -> [w223]
          tunnel: ["stop"] -> w116
          tunnel: [w187] -> w115
          tunnel: w114 -> [w182]
          tunnel: w113 -> [w180]
          shift-right: [w159] -> _
          shift-left: i32[] [] -> [w150]
          tunnel: w111 -> [w149]
          tunnel: w110 -> [w142]
          tunnel: [w141] -> w109
          stop <- w186 stop-if-true
          n19 = flat-sequence {
            tunnel: w289 -> [w393]
            tunnel: w328 -> [w394]
            tunnel: w332 -> [w395]
            tunnel: w334 -> [w396]
            tunnel: w335 -> [w397]
            tunnel: w336 -> [w398]
            tunnel: w363 -> [w399]
            tunnel: w364 -> [w400]
            tunnel: w378 -> [w401]
            tunnel: w379 -> [w402]
            tunnel: w380 -> [w403]
            tunnel: [w403] -> w288
            tunnel: [w402] -> w287
            tunnel: [w401] -> w286
            tunnel: [w400] -> w285
            tunnel: [w399] -> w284
            tunnel: [w398] -> w283
            tunnel: [w397] -> w282
            tunnel: [w396] -> w281
            tunnel: [w395] -> w280
            tunnel: [w394] -> w279
            tunnel: [w393] -> w278
            tunnel: [w392] -> w260
            tunnel: [w391] -> w246
            tunnel: w245 -> [w391]
            tunnel: [w390] -> w242
            tunnel: w241 -> [w390]
            tunnel: [w389] -> w230
            tunnel: w229 -> [w389]
            tunnel: [w388] -> w228
            tunnel: w227 -> [w388]
            tunnel: [w387] -> w226
            tunnel: w225 -> [w387]
            tunnel: [w386] -> w224
            tunnel: w223 -> [w386]
            tunnel: [w385] -> w183
            tunnel: w182 -> [w385]
            tunnel: [w384] -> w181
            tunnel: w180 -> [w384]
            tunnel: [w383] -> w151
            tunnel: w150 -> [w383]
            tunnel: w149 -> [w382]
            tunnel: [w382] -> w148
            tunnel: [w381] -> w143
            tunnel: w142 -> [w381]
            tunnel: [w429] -> w377
            tunnel: [w428] -> w375
            tunnel: [w424] -> w373
            tunnel: [w423] -> w368
            tunnel: [w422] -> w366
            tunnel: [w421] -> w333
            tunnel: [w420] -> w329
            tunnel: [w419] -> w309
            tunnel: [w418] -> w306
            tunnel: [w417] -> w304
            tunnel: [w416] -> w290
            tunnel: w288 -> [w429]
            tunnel: w287 -> [w428]
            tunnel: w286 -> [w427]
            tunnel: w285 -> [w423]
            tunnel: w284 -> [w422]
            tunnel: w283 -> [w419]
            tunnel: w282 -> [w418]
            tunnel: w281 -> [w417]
            tunnel: w280 -> [w421]
            tunnel: w279 -> [w420]
            tunnel: w278 -> [w416]
            tunnel: [w415] -> w261
            tunnel: w260 -> [w415]
            tunnel: w246 -> [w413]
            tunnel: [w413] -> w243
            tunnel: w242 -> [w414]
            tunnel: [w414] -> w239
            tunnel: w230 -> [w412]
            tunnel: w228 -> [w411]
            tunnel: w226 -> [w410]
            tunnel: w224 -> [w409]
            tunnel: [w412] -> w222
            tunnel: [w411] -> w218
            tunnel: [w410] -> w215
            tunnel: [w409] -> w214
            tunnel: w183 -> [w408]
            tunnel: w181 -> [w407]
            tunnel: [w408] -> w178
            tunnel: [w407] -> w176
            tunnel: [w406] -> w152
            tunnel: w151 -> [w406]
            tunnel: w148 -> [w404]
            tunnel: [w404] -> w147
            tunnel: [w405] -> w144
            tunnel: w143 -> [w405]
            tunnel: w377 -> [w1045]
            tunnel: [w1045] -> w376
            tunnel: w375 -> [w1044]
            tunnel: [w1044] -> w374
            tunnel: w373 -> [w1040]
            tunnel: [w1040] -> w372
            tunnel: w371 -> [w1041]
            tunnel: [w1041] -> w370
            tunnel: [w1041] -> w369
            tunnel: w368 -> [w1043]
            tunnel: [w1043] -> w367
            tunnel: w366 -> [w1042]
            tunnel: [w1042] -> w365
            tunnel: [w1041] -> w362
            tunnel: [w1041] -> w348
            tunnel: w333 -> [w1039]
            tunnel: [w1039] -> w331
            tunnel: w329 -> [w1038]
            tunnel: [w1038] -> w326
            tunnel: [w1037] -> w310
            tunnel: w309 -> [w1037]
            tunnel: [w1036] -> w307
            tunnel: w306 -> [w1036]
            tunnel: [w1035] -> w305
            tunnel: w304 -> [w1035]
            tunnel: [w1034] -> w291
            tunnel: w290 -> [w1034]
            tunnel: [w1033] -> w262
            tunnel: w261 -> [w1033]
            tunnel: [w1032] -> w244
            tunnel: w243 -> [w1032]
            tunnel: [w1031] -> w240
            tunnel: w239 -> [w1031]
            tunnel: w222 -> [w1030]
            tunnel: [w1030] -> w221
            tunnel: [w1029] -> w219
            tunnel: w218 -> [w1029]
            tunnel: [w1028] -> w217
            tunnel: w215 -> [w1028]
            tunnel: w214 -> [w1027]
            tunnel: [w1027] -> w213
            tunnel: [w1026] -> w179
            tunnel: w178 -> [w1026]
            tunnel: [w1025] -> w177
            tunnel: w176 -> [w1025]
            tunnel: [w1024] -> w153
            tunnel: w152 -> [w1024]
            tunnel: w147 -> [w1023]
            tunnel: [w1023] -> w146
            tunnel: [w1022] -> w145
            tunnel: w144 -> [w1022]
            tunnel: [w1074] -> w347
            tunnel: w376 -> [w1103]
            tunnel: w374 -> [w1102]
            tunnel: w372 -> [w1099]
            tunnel: w370 -> [w1098]
            tunnel: w369 -> [w1097]
            tunnel: w367 -> [w1087]
            tunnel: w365 -> [w1086]
            tunnel: w362 -> [w1088]
            tunnel: [w1084] -> w346
            tunnel: [w1085] -> w345
            tunnel: [w1096] -> w344
            tunnel: [w1095] -> w343
            tunnel: [w1094] -> w342
            tunnel: [w1093] -> w341
            tunnel: w348 -> [w1083]
            tunnel: [w1082] -> w340
            tunnel: [w1081] -> w339
            tunnel: [w1065] -> w338
            tunnel: [w1080] -> w337
            tunnel: w331 -> [w1079]
            tunnel: [w1079] -> w330
            tunnel: [w1078] -> w327
            tunnel: w326 -> [w1078]
            tunnel: w310 -> [w1077]
            tunnel: [w1077] -> w308
            tunnel: w307 -> [w1076]
            tunnel: w305 -> [w1075]
            tunnel: [w1076] -> w303
            tunnel: [w1075] -> w302
            tunnel: w291 -> [w1073]
            tunnel: [w1069] -> w263
            tunnel: w262 -> [w1069]
            tunnel: w244 -> [w1067]
            tunnel: w240 -> [w1066]
            tunnel: [w1060] -> w238
            tunnel: [w1065] -> w237
            tunnel: [w1063] -> w236
            tunnel: [w1061] -> w235
            tunnel: w221 -> [w1064]
            tunnel: [w1064] -> w220
            tunnel: w219 -> [w1063]
            tunnel: w217 -> [w1062]
            tunnel: [w1062] -> w216
            tunnel: w213 -> [w1061]
            tunnel: [w1060] -> w191
            tunnel: [w1059] -> w188
            tunnel: w179 -> [w1058]
            tunnel: w177 -> [w1057]
            tunnel: [w1054] -> w172
            tunnel: [w1052] -> w171
            tunnel: [w1054] -> w170
            tunnel: [w1053] -> w166
            tunnel: [w1052] -> w163
            tunnel: [w1051] -> w160
            tunnel: [w1050] -> w154
            tunnel: w153 -> [w1050]
            tunnel: w146 -> [w1049]
            tunnel: w145 -> [w1048]
            tunnel: [w1047] -> w141
            tunnel: w347 -> [w1342]
            tunnel: [w1339] -> w321
            tunnel: w346 -> [w1355]
            tunnel: [w1355] -> w320
            tunnel: w345 -> [w1354]
            tunnel: [w1354] -> w319
            tunnel: w344 -> [w1353]
            tunnel: [w1353] -> w318
            tunnel: w343 -> [w1352]
            tunnel: [w1352] -> w317
            tunnel: w342 -> [w1351]
            tunnel: [w1351] -> w316
            tunnel: w341 -> [w1350]
            tunnel: [w1350] -> w315
            tunnel: [w1343] -> w314
            tunnel: w340 -> [w1336]
            tunnel: w339 -> [w1344]
            tunnel: w338 -> [w1343]
            tunnel: w337 -> [w1345]
            tunnel: [w1342] -> w313
            tunnel: w330 -> [w1341]
            tunnel: w327 -> [w1340]
            tunnel: [w1338] -> w312
            tunnel: [w1326] -> w311
            tunnel: w308 -> [w1337]
            tunnel: w303 -> [w1334]
            tunnel: w302 -> [w1333]
            tunnel: [w1335] -> w299
            tunnel: [w1332] -> w296
            tunnel: [w1331] -> w293
            tunnel: [w1327] -> w292
            tunnel: [w1325] -> w264
            tunnel: w263 -> [w1325]
            tunnel: w238 -> [w1324]
            tunnel: w237 -> [w1323]
            tunnel: w236 -> [w1322]
            tunnel: w235 -> [w1320]
            tunnel: [w1318] -> w234
            tunnel: [w1317] -> w233
            tunnel: [w1316] -> w232
            tunnel: [w1315] -> w231
            tunnel: w220 -> [w1319]
            tunnel: w216 -> [w1321]
            tunnel: [w1318] -> w212
            tunnel: [w1317] -> w211
            tunnel: [w1316] -> w210
            tunnel: [w1315] -> w209
            tunnel: [w1314] -> w192
            tunnel: w191 -> [w1314]
            tunnel: [w1313] -> w189
            tunnel: w188 -> [w1313]
            tunnel: w172 -> [w1312]
            tunnel: w171 -> [w1311]
            tunnel: w170 -> [w1310]
            tunnel: [w1310] -> w169
            tunnel: [w1309] -> w167
            tunnel: w166 -> [w1309]
            tunnel: w163 -> [w1308]
            tunnel: [w1308] -> w162
            tunnel: [w1307] -> w161
            tunnel: w160 -> [w1307]
            tunnel: [w1306] -> w155
            tunnel: w154 -> [w1306]
            tunnel: w321 -> [w1394]
            tunnel: [w1401] -> w361
            tunnel: [w1400] -> w360
            tunnel: w320 -> [w1400]
            tunnel: [w1395] -> w357
            tunnel: w319 -> [w1395]
            tunnel: [w1399] -> w355
            tunnel: w318 -> [w1399]
            tunnel: [w1398] -> w353
            tunnel: w317 -> [w1398]
            tunnel: [w1397] -> w351
            tunnel: w316 -> [w1397]
            tunnel: [w1396] -> w349
            tunnel: w315 -> [w1396]
            tunnel: w314 -> [w1383]
            tunnel: w313 -> [w1384]
            tunnel: w312 -> [w1362]
            tunnel: [w1362] -> w324
            tunnel: w311 -> [w1385]
            tunnel: [w1385] -> w322
            tunnel: [w1387] -> w300
            tunnel: w299 -> [w1387]
            tunnel: [w1388] -> w297
            tunnel: w296 -> [w1388]
            tunnel: [w1389] -> w294
            tunnel: w293 -> [w1389]
            tunnel: w292 -> [w1393]
            tunnel: [w1382] -> w265
            tunnel: w264 -> [w1382]
            tunnel: w234 -> [w1381]
            tunnel: w233 -> [w1380]
            tunnel: w232 -> [w1379]
            tunnel: w231 -> [w1378]
            tunnel: w212 -> [w1377]
            tunnel: w211 -> [w1376]
            tunnel: w210 -> [w1375]
            tunnel: w209 -> [w1374]
            tunnel: [w1377] -> w207
            tunnel: [w1376] -> w205
            tunnel: [w1375] -> w203
            tunnel: [w1374] -> w201
            tunnel: w192 -> [w1373]
            tunnel: [w1372] -> w190
            tunnel: w189 -> [w1372]
            tunnel: w169 -> [w1369]
            tunnel: [w1368] -> w168
            tunnel: w167 -> [w1368]
            tunnel: w162 -> [w1367]
            tunnel: w161 -> [w1359]
            tunnel: [w1361] -> w156
            tunnel: w155 -> [w1360]
            tunnel: w361 -> [w1419]
            tunnel: w360 -> [w1433]
            tunnel: w357 -> [w1427]
            tunnel: w355 -> [w1432]
            tunnel: w353 -> [w1429]
            tunnel: w351 -> [w1431]
            tunnel: w349 -> [w1430]
            tunnel: w324 -> [w1424]
            tunnel: w322 -> [w1423]
            tunnel: w300 -> [w1422]
            tunnel: w297 -> [w1421]
            tunnel: w294 -> [w1420]
            tunnel: [w1413] -> w185
            tunnel: [w1433] -> w277
            tunnel: [w1427] -> w276
            tunnel: [w1432] -> w275
            tunnel: [w1429] -> w274
            tunnel: [w1431] -> w273
            tunnel: [w1430] -> w272
            tunnel: [w1424] -> w271
            tunnel: [w1423] -> w270
            tunnel: [w1422] -> w269
            tunnel: [w1421] -> w268
            tunnel: [w1420] -> w267
            tunnel: [w1418] -> w266
            tunnel: w265 -> [w1418]
            tunnel: [w1417] -> w208
            tunnel: w207 -> [w1417]
            tunnel: [w1416] -> w206
            tunnel: w205 -> [w1416]
            tunnel: [w1415] -> w204
            tunnel: w203 -> [w1415]
            tunnel: [w1414] -> w202
            tunnel: w201 -> [w1414]
            tunnel: w190 -> [w1412]
            tunnel: [w1411] -> w175
            tunnel: [w1410] -> w174
            tunnel: w168 -> [w1409]
            tunnel: [w1408] -> w165
            tunnel: [w1407] -> w164
            tunnel: [w1402] -> w157
            tunnel: w156 -> [w1402]
            tunnel: w277 -> [w1481]
            tunnel: w276 -> [w1480]
            tunnel: w275 -> [w1479]
            tunnel: w274 -> [w1478]
            tunnel: w273 -> [w1477]
            tunnel: w272 -> [w1476]
            tunnel: w271 -> [w1475]
            tunnel: w270 -> [w1474]
            tunnel: w269 -> [w1473]
            tunnel: w268 -> [w1472]
            tunnel: w267 -> [w1471]
            tunnel: w266 -> [w1467]
            tunnel: [w1481] -> w259
            tunnel: [w1480] -> w258
            tunnel: [w1479] -> w257
            tunnel: [w1478] -> w256
            tunnel: [w1477] -> w255
            tunnel: [w1476] -> w254
            tunnel: [w1475] -> w253
            tunnel: [w1474] -> w252
            tunnel: [w1473] -> w251
            tunnel: [w1472] -> w250
            tunnel: [w1471] -> w249
            tunnel: [w1467] -> w248
            tunnel: [w1466] -> w247
            tunnel: w208 -> [w1464]
            tunnel: w206 -> [w1463]
            tunnel: w204 -> [w1462]
            tunnel: w202 -> [w1461]
            tunnel: [w1464] -> w200
            tunnel: [w1463] -> w198
            tunnel: [w1462] -> w196
            tunnel: [w1461] -> w194
            tunnel: w175 -> [w1460]
            tunnel: w174 -> [w1459]
            tunnel: [w1454] -> w173
            tunnel: w165 -> [w1453]
            tunnel: w164 -> [w1452]
            tunnel: [w1451] -> w158
            tunnel: w157 -> [w1451]
            tunnel: [w1493] -> w295
            tunnel: [w1494] -> w298
            tunnel: [w1495] -> w301
            tunnel: [w1496] -> w323
            tunnel: [w1497] -> w325
            tunnel: [w1498] -> w350
            tunnel: [w1499] -> w352
            tunnel: [w1500] -> w354
            tunnel: [w1501] -> w356
            tunnel: [w1502] -> w358
            tunnel: [w1503] -> w359
            tunnel: w259 -> [w1503]
            tunnel: w258 -> [w1502]
            tunnel: w257 -> [w1501]
            tunnel: w256 -> [w1500]
            tunnel: w255 -> [w1499]
            tunnel: w254 -> [w1498]
            tunnel: w253 -> [w1497]
            tunnel: w252 -> [w1496]
            tunnel: w251 -> [w1495]
            tunnel: w250 -> [w1494]
            tunnel: w249 -> [w1493]
            tunnel: w248 -> [w1489]
            tunnel: w247 -> [w1488]
            tunnel: [w1487] -> w199
            tunnel: w200 -> [w1487]
            tunnel: [w1486] -> w197
            tunnel: w198 -> [w1486]
            tunnel: [w1485] -> w195
            tunnel: w196 -> [w1485]
            tunnel: [w1484] -> w193
            tunnel: w194 -> [w1484]
            tunnel: [w1483] -> w187
            tunnel: w173 -> [w1483]
            tunnel: [w1482] -> w159
            tunnel: w158 -> [w1482]
            frame #0 {
              n20 = Tick Count (ms)() -> (millisecond timer value=w392:u32)
            }
            frame #1 {
              n21 = while {
                tunnel: w427 -> [w435]
                tunnel: [w434] -> w426
                tunnel: [w433] -> w425
                tunnel: w413 -> [w431]
                tunnel: w404 -> [w430]
                stop <- w436 stop-if-true
                n22 = event shown="[1] \"Setpoint  START\": Value Change" {
                  selector: _ -> [_ _ _ _ _ _ _ _ _ _ _ _ _ _ _]
                  dyn-events: _ -> [_ _ _ _ _ _ _ _ _ _ _ _ _ _ _]
                  timeout: 1 -> [_ _ _ _ _ _ _ _ _ _ _ _ _ _ _]
                  tunnel: [TRUE ("Set Gauge to Zero") w444 w493 w514 w540 w575 w631 w682 w761 w832 "Set Gauge to Zero" _ _ "Get SetPoint" _] -> w436
                  tunnel: w435 -> [w440 w443 w490 w512 w536 w574 w627 w680 w759 w830 w907 w929 w937 w1009 _]
                  tunnel: [w439 w442 w489 w511 w538 w572 w629 w679 w758 w829 w906 w928 w936 w1008 _] -> w434
                  tunnel: [w438 w441 w488 w510 w537 w573 w628 w678 w757 w828 w905 w927 w935 w1007 _] -> w433
                  tunnel: w431 -> [_ _ _ _ _ _ _ _ _ _ w903 _ _ _ _]
                  tunnel: w430 -> [_ _ _ _ _ _ _ _ _ _ _ _ _ _ w1021]
                  event Timeout {
                    n23 = event-data() -> ()  [unwired: 1 in, 1 out]
                    n24 = Unbundle(w440) -> ("VISA resource name out"=w439:refnum<visa-resource-name>, "error out"=w438:errorcluster)  [unwired: 2 out]
                  }
                  event "Setpoint\n START": Value Change {
                    n25 = event-data() -> ()  [unwired: 1 in, 1 out]
                    n26 = stacked-sequence {
                      tunnel: w443 -> [_ w450 _]
                      tunnel: [_ w449 _] -> w441
                      tunnel: [_ w448 _] -> w442
                      frame #0 {
                        n27 = property on="Setpoint\n START" class="Bool"("Blinking"=TRUE) -> ()  [unwired: 2 in, 2 out]
                        n28 = property on="ON" class="Bool (strict)"("Blinking"=FALSE) -> ()  [unwired: 2 in, 2 out]
                      }
                      frame #1 {
                        n29 = for {
                          N: 2 -> [_]
                          tunnel: w450 -> [w454]
                          tunnel: [w453] -> w449
                          tunnel: [w452] -> w448
                          i -> [w456]
                          n30 = flat-sequence {
                            tunnel: [w459] -> w455
                            tunnel: w456 -> [w458]
                            tunnel: [w477] -> w457
                            tunnel: w455 -> [w476]
                            tunnel: w454 -> [w478]
                            tunnel: [w475] -> w453
                            tunnel: [w474] -> w452
                            tunnel: w457 -> [w484]
                            tunnel: w456 -> [w483]
                            frame #0 {
                              n31 = case shown="1" w458 {
                                tunnel: [w468 w470] -> w459
                                frame 0, Default {
                                n32 = Multiply(x=10.0, y="SP 1 input (°C)") -> (x*y=w465:dbl)
                                n33 = local read "RAM"() -> (w463:bool)
                                n34 = Number To Hexadecimal String(1:i16 5 ("width (-)"), 2:w465) -> (0:w467:string)
                                n35 = Select(t="*P012", s=w463, f="*P012") -> (s? t:f=w460:string)
                                n36 = Concatenate Strings(w460, w467) -> (w468:string)
                                }
                                frame 1 {
                                n37 = local read "RAM"() -> (w473:bool)
                                n38 = Select(t="*G01", s=w473, f="*R01") -> (s? t:f=w470:string)
                                }
                              }
                            }
                            frame #1 {
                              n39 = Unbundle(w478) -> ("VISA resource name out"=w479:refnum<visa-resource-name>, "error out"=w481:errorcluster, "Delay (ms)"=w480:u32, "Write/\nRead"=w482:bool)
                              n40 = call "I3252_Comm_Interface.vi"("VISA resource name in"=w479, "error in"=w481, "Delay (ms)"=w480, "Write"=w482, "String to Write"=w476, "Read"=w482) -> ("VISA resource name out"=w474:refnum<visa-resource-name>, "error out"=w475:errorcluster, "Read String"=w477:string)  [unwired: 2 in]
                            }
                            frame #2 {
                              n41 = case shown="1" w483 {
                                tunnel: w484 -> [_ w486]
                                frame 0, Default {
                                }
                                frame 1 {
                                n42 = call "I3252_Edit_Setpoint.vi"("Read String"=w486) -> ("Setpoint is"=→"SP 1 is (°C)":dbl)
                                }
                              }
                            }
                          }
                        }
                      }
                      frame #2 {
                        n43 = property on="Setpoint\n START" class="Bool"("Blinking"=FALSE) -> ()  [unwired: 2 in, 2 out]
                      }
                    }
                    n44 = Not(x="Setpoint\n START") -> (.not. x?=w444:bool)
                  }
                  event "Standby": Value Change {
                    n45 = event-data() -> ()  [unwired: 1 in, 1 out]
                    n46 = flat-sequence {
                      tunnel: [w501] -> w491
                      tunnel: w491 -> [w505]
                      tunnel: w490 -> [w504]
                      tunnel: [w503] -> w488
                      tunnel: [w502] -> w489
                      frame #0 {
                        n47 = local read "Standby"() -> (w494:bool)
                        n48 = Select(t=TRUE, s=w494, f=FALSE) -> (s? t:f=w497:bool)
                        n49 = property on="Standby" class="Bool (strict)"("Blinking"=w497) -> ()  [unwired: 2 in, 2 out]
                      }
                      frame #1 {
                        n50 = local read "Standby"() -> (w499:bool)
                        n51 = Select(t="*D03", s=w499, f="*E03") -> (s? t:f=w501:string)
                      }
                      frame #2 {
                        n52 = Unbundle(w504) -> ("VISA resource name out"=w506:refnum<visa-resource-name>, "error out"=w508:errorcluster, "Delay (ms)"=w507:u32, "Write/\nRead"=w509:bool)
                        n53 = call "I3252_Comm_Interface.vi"("VISA resource name in"=w506, "error in"=w508, "Delay (ms)"=w507, "Write"=w509, "String to Write"=w505, "Read"=w509) -> ("VISA resource name out"=w502:refnum<visa-resource-name>, "error out"=w503:errorcluster)  [unwired: 2 in, 1 out]
                      }
                    }
                    n54 = Not(x="Standby") -> (.not. x?=w493:bool)
                  }
                  event "Set Command": Value Change {
                    n55 = event-data() -> ()  [unwired: 1 in, 1 out]
                    n56 = stacked-sequence {
                      tunnel: w512 -> [_ w519 _]
                      tunnel: [_ w518 _] -> w511
                      tunnel: [_ w517 _] -> w510
                      frame #0 {
                        n57 = property on="Set Command" class="Bool"("Blinking"=TRUE) -> ()  [unwired: 2 in, 2 out]
                        n58 = property on="ON" class="Bool (strict)"("Blinking"=FALSE) -> ()  [unwired: 2 in, 2 out]
                      }
                      frame #1 {
                        n59 = flat-sequence {
                          tunnel: [w524] -> w521
                          tunnel: [w527] -> w520
                          tunnel: w521 -> [w528]
                          tunnel: w519 -> [w529]
                          tunnel: [w526] -> w518
                          tunnel: [w525] -> _
                          tunnel: [w525] -> w517
                          tunnel: w520 -> [w534]
                          frame #0 {
                            n60 = Concatenate Strings("*", "Command input") -> (w524:string)
                          }
                          frame #1 {
                            n61 = Unbundle(w529) -> ("VISA resource name out"=w533:refnum<visa-resource-name>, "error out"=w531:errorcluster, "Delay (ms)"=w532:u32, "Write/\nRead"=w530:bool)
                            n62 = call "I3252_Comm_Interface.vi"("VISA resource name in"=w533, "error in"=w531, "Delay (ms)"=w532, "Write"=w530, "String to Write"=w528, "Read"=w530) -> ("VISA resource name out"=w526:refnum<visa-resource-name>, "error out"=w525:errorcluster, "Read String"=w527:string)  [unwired: 2 in]
                          }
                          frame #2 {
                            "Command output" <- w534
                          }
                        }
                      }
                      frame #2 {
                        n63 = property on="Set Command" class="Bool"("Blinking"=FALSE) -> ()  [unwired: 2 in, 2 out]
                      }
                    }
                    n64 = Not(x="Set Command") -> (.not. x?=w514:bool)
                  }
                  event "Reset\nSTOPP": Value Change {
                    n65 = event-data() -> ()  [unwired: 1 in, 1 out]
                    n66 = stacked-sequence {
                      tunnel: [_ w547 _] -> w537
                      tunnel: [_ w546 _] -> w538
                      tunnel: w536 -> [_ w544 _]
                      frame #0 {
                        n67 = property on="Reset\nSTOPP" class="Bool"("Blinking"=FALSE) -> ()  [unwired: 2 in, 2 out]
                        n68 = property on="ON" class="Bool (strict)"("Blinking"=FALSE) -> ()  [unwired: 2 in, 2 out]
                      }
                      frame #1 {
                        n69 = for {
                          N: 2 -> [_]
                          tunnel: [w553] -> w547
                          tunnel: [w552] -> w546
                          tunnel: w544 -> [w551]
                          i -> [w549]
                          n70 = flat-sequence {
                            tunnel: w549 -> [w555]
                            tunnel: [w554] -> w550
                            tunnel: [w560] -> w553
                            tunnel: [w561] -> w552
                            tunnel: w551 -> [w562]
                            tunnel: w550 -> [w559]
                            tunnel: [w558] -> w548
                            tunnel: w549 -> [w568]
                            tunnel: w548 -> [w567]
                            frame #0 {
                              n71 = case shown="0, Default" w555 {
                                tunnel: ["*Z02" "*G01"] -> w554
                                frame 0, Default {
                                }
                                frame 1 {
                                }
                              }
                            }
                            frame #1 {
                              n72 = Unbundle(w562) -> ("VISA resource name out"=w563:refnum<visa-resource-name>, "error out"=w565:errorcluster, "Delay (ms)"=w564:u32, "Write/\nRead"=w566:bool)
                              n73 = call "I3252_Comm_Interface.vi"("VISA resource name in"=w563, "error in"=w565, "Delay (ms)"=w564, "Write"=w566, "String to Write"=w559, "Read"=w566) -> ("VISA resource name out"=w561:refnum<visa-resource-name>, "error out"=w560:errorcluster, "Read String"=w558:string)  [unwired: 2 in]
                            }
                            frame #2 {
                              n74 = case shown="0, Default" w568 {
                                tunnel: w567 -> [_ w570]
                                frame 0, Default {
                                }
                                frame 1 {
                                n75 = call "I3252_Edit_Setpoint.vi"("Read String"=w570) -> ("Setpoint is"=w569:dbl)
                                n76 = local write "SP 1 is (°C)"(w569) -> ()
                                }
                              }
                            }
                          }
                        }
                        n77 = Wait (ms)(milliseconds to wait=u32 4000) -> ()  [unwired: 1 out]
                      }
                      frame #2 {
                        n78 = property on="Reset\nSTOPP" class="Bool"("Blinking"=FALSE) -> ()  [unwired: 2 in, 2 out]
                      }
                    }
                    n79 = Not(x="Reset\nSTOPP") -> (.not. x?=w540:bool)
                  }
                  event "Auto Tune": Value Change {
                    n80 = event-data() -> ()  [unwired: 1 in, 1 out]
                    n81 = stacked-sequence {
                      tunnel: w574 -> [_ w581 w626]
                      tunnel: [_ w580 _] -> w573
                      tunnel: [_ w579 _] -> w572
                      frame #0 {
                        n82 = property on="Auto Tune" class="Bool"("Blinking"=TRUE) -> ()  [unwired: 2 in, 2 out]
                        n83 = property on="ON" class="Bool (strict)"("Blinking"=FALSE) -> ()  [unwired: 2 in, 2 out]
                      }
                      frame #1 {
                        n84 = for {
                          N: 4 -> [_]
                          tunnel: [w586] -> w579
                          tunnel: [w585] -> w580
                          tunnel: w581 -> [w584]
                          i -> [w589]
                          n85 = flat-sequence {
                            tunnel: w589 -> [w591]
                            tunnel: [w590] -> w587
                            tunnel: w587 -> [w606]
                            tunnel: [w605] -> w588
                            tunnel: [w608] -> w586
                            tunnel: [w607] -> w585
                            tunnel: w584 -> [w604]
                            tunnel: w589 -> [w614]
                            tunnel: w588 -> [w613]
                            frame #0 {
                              n86 = case shown="2" w591 {
                                tunnel: ["*V01" w594 "*W0C35" "*Z02"] -> w590
                                frame 0, Default {
                                }
                                frame 1 {
                                n87 = local read "(°C)"() -> (w593:dbl)
                                n88 = Add(x=20.0, y=w593) -> (x+y=w600:dbl)
                                n89 = Multiply(x=10.0, y=w600) -> (x*y=w597:dbl)
                                n90 = Number To Hexadecimal String(1:i16 5 ("width (-)"), 2:w597) -> (0:w596:string)
                                n91 = Concatenate Strings("*W012", w596) -> (w594:string)
                                }
                                frame 2 {
                                # "35 hex = \n00110101 bin"
                                }
                                frame 3 {
                                }
                              }
                            }
                            frame #1 {
                              n92 = Unbundle(w604) -> ("VISA resource name out"=w612:refnum<visa-resource-name>, "error out"=w610:errorcluster, "Delay (ms)"=w611:u32, "Write/\nRead"=w609:bool)
                              n93 = call "I3252_Comm_Interface.vi"("VISA resource name in"=w612, "error in"=w610, "Delay (ms)"=w611, "Write"=w609, "String to Write"=w606, "Read"=w609) -> ("VISA resource name out"=w608:refnum<visa-resource-name>, "error out"=w607:errorcluster, "Read String"=w605:string)  [unwired: 2 in]
                            }
                            frame #2 {
                              n94 = case shown="0, Default" w614 {
                                tunnel: w613 -> [w616]
                                frame 0, Default {
                                n95 = call <vilib>:"Space Constant.vi"() -> ("String"=w619:string)
                                n96 = Search/Split String(string=w616, search string/char (-)=w619) -> (match + rest of string=w618:string)  [unwired: 1 in, 2 out]
                                n97 = Fract/Exp String To Number(use system decimal point (T)=FALSE, string=w618) -> (number=w615:dbl)  [unwired: 2 in, 1 out]
                                n98 = local write "(°C)"(w615) -> ()
                                }
                              }
                            }
                          }
                        }
                        n99 = Wait (ms)(milliseconds to wait=u32 45000) -> ()  [unwired: 1 out]
                      }
                      frame #2 {
                        n100 = Unbundle(w626) -> ("VISA resource name out"=w625:refnum<visa-resource-name>, "error out"=w623:errorcluster, "Delay (ms)"=w624:u32, "Write/\nRead"=w622:bool)
                        n101 = property on="Auto Tune" class="Bool"("Blinking"=FALSE) -> ()  [unwired: 2 in, 2 out]
                        n102 = call "I3252_Comm_Interface.vi"("VISA resource name in"=w625, "error in"=w623, "Delay (ms)"=w624, "Write"=w622, "String to Write"="*W01200000", "Read"=w622) -> ()  [unwired: 2 in, 3 out]
                      }
                    }
                    n103 = Not(x="Auto Tune") -> (.not. x?=w575:bool)
                  }
                  event "Write LOW/HI": Value Change {
                    n104 = event-data() -> ()  [unwired: 1 in, 1 out]
                    n105 = stacked-sequence {
                      tunnel: [_ w636 _] -> w629
                      tunnel: [_ w635 _] -> w628
                      tunnel: w627 -> [_ w634 _]
                      frame #0 {
                        n106 = property on="Write LOW/HI" class="Bool"("Blinking"=TRUE) -> ()  [unwired: 2 in, 2 out]
                        n107 = property on="ON" class="Bool (strict)"("Blinking"=FALSE) -> ()  [unwired: 2 in, 2 out]
                      }
                      frame #1 {
                        n108 = for {
                          N: 4 -> [_]
                          tunnel: [w640] -> w636
                          tunnel: [w639] -> w635
                          tunnel: w634 -> [w638]
                          i -> [w642]
                          n109 = flat-sequence {
                            tunnel: w642 -> [w644]
                            tunnel: [w645] -> w641
                            tunnel: w641 -> [w659]
                            tunnel: [w660] -> w643
                            tunnel: [w662] -> w640
                            tunnel: [w661] -> w639
                            tunnel: w638 -> [w658]
                            tunnel: w643 -> [w668]
                            tunnel: w642 -> [w667]
                            frame #0 {
                              n110 = case shown="1" w644 {
                                tunnel: [w647 w653 "*R27" "*R28"] -> w645
                                frame 0, Default {
                                n111 = Number To Hexadecimal String(1:i16 2 ("width (-)"), 2:"% LOW Sollwert") -> (0:w648:string)
                                n112 = Concatenate Strings("*W27", w648) -> (w647:string)
                                }
                                frame 1 {
                                n113 = Number To Hexadecimal String(1:i16 2 ("width (-)"), 2:"% High Sollwert") -> (0:w654:string)
                                n114 = Concatenate Strings("*W28", w654) -> (w653:string)
                                }
                                frame 2 {
                                }
                                frame 3 {
                                }
                              }
                            }
                            frame #1 {
                              n115 = Unbundle(w658) -> ("VISA resource name out"=w666:refnum<visa-resource-name>, "error out"=w664:errorcluster, "Delay (ms)"=w665:u32, "Write/\nRead"=w663:bool)
                              n116 = call "I3252_Comm_Interface.vi"("VISA resource name in"=w666, "error in"=w664, "Delay (ms)"=w665, "Write"=w663, "String to Write"=w659, "Read"=w663) -> ("VISA resource name out"=w662:refnum<visa-resource-name>, "error out"=w661:errorcluster, "Read String"=w660:string)  [unwired: 2 in]
                            }
                            frame #2 {
                              n117 = case shown="0, Default" w667 {
                                tunnel: w668 -> [_ w672 w676]
                                frame 0, Default {
                                }
                                frame 2 {
                                n118 = String Subset(string=w672, offset (0)=3) -> (substring=w670:string)  [unwired: 1 in]
                                n119 = Hexadecimal String To Number(string=w670) -> (number=→"% LOW Istwert":u32)  [unwired: 2 in, 1 out]
                                }
                                frame 3 {
                                n120 = String Subset(string=w676, offset (0)=3) -> (substring=w674:string)  [unwired: 1 in]
                                n121 = Hexadecimal String To Number(string=w674) -> (number=→"% HIGH Istwert":u32)  [unwired: 2 in, 1 out]
                                }
                              }
                            }
                          }
                        }
                      }
                      frame #2 {
                        n122 = property on="Write LOW/HI" class="Bool"("Blinking"=FALSE) -> ()  [unwired: 2 in, 2 out]
                      }
                    }
                    n123 = Not(x="Write LOW/HI") -> (.not. x?=w631:bool)
                  }
                  event "Set PID": Value Change {
                    n124 = event-data() -> ()  [unwired: 1 in, 1 out]
                    n125 = stacked-sequence {
                      tunnel: w680 -> [_ w687 _]
                      tunnel: [_ w686 _] -> w679
                      tunnel: [_ w685 _] -> w678
                      frame #0 {
                        n126 = property on="Set PID" class="Bool"("Blinking"=TRUE) -> ()  [unwired: 2 in, 2 out]
                        n127 = property on="ON" class="Bool (strict)"("Blinking"=FALSE) -> ()  [unwired: 2 in, 2 out]
                      }
                      frame #1 {
                        n128 = for {
                          N: 6 -> [_]
                          tunnel: w687 -> [w691]
                          tunnel: [w690] -> w686
                          tunnel: [w689] -> w685
                          i -> [w693]
                          n129 = flat-sequence {
                            tunnel: w693 -> [w695]
                            tunnel: [w696] -> w692
                            tunnel: w692 -> [w737]
                            tunnel: [w733] -> w694
                            tunnel: w691 -> [w736]
                            tunnel: [w735] -> w689
                            tunnel: [w734] -> w690
                            tunnel: w694 -> [w743]
                            tunnel: w693 -> [w742]
                            frame #0 {
                              n130 = case shown="0, Default" w695 {
                                tunnel: [w703 w711 w719 w721 w725 w729] -> w696
                                frame 0, Default {
                                n131 = local read "RAM"() -> (w697:bool)
                                n132 = Number To Hexadecimal String(1:i16 4 ("width (-)"), 2:"P (PB1) Sollwert") -> (0:w704:string)
                                n133 = Select(t="*P17", s=w697, f="*W17") -> (s? t:f=w698:string)
                                n134 = Concatenate Strings(w698, w704) -> (w703:string)
                                }
                                frame 1 {
                                n135 = local read "RAM"() -> (w705:bool)
                                n136 = Number To Hexadecimal String(1:i16 4 ("width (-)"), 2:"I ( Reset1) Sollwert") -> (0:w712:string)
                                n137 = Select(t="*P18", s=w705, f="*W18") -> (s? t:f=w707:string)
                                n138 = Concatenate Strings(w707, w712) -> (w711:string)
                                }
                                frame 2 {
                                n139 = local read "RAM"() -> (w714:bool)
                                n140 = Number To Hexadecimal String(1:i16 4 ("width (-)"), 2:"D (Rate) Sollwert") -> (0:w720:string)
                                n141 = Select(t="*P19", s=w714, f="*W19") -> (s? t:f=w715:string)
                                n142 = Concatenate Strings(w715, w720) -> (w719:string)
                                }
                                frame 3 {
                                n143 = local read "RAM"() -> (w724:bool)
                                n144 = Select(t="*G17", s=w724, f="*R17") -> (s? t:f=w721:string)
                                }
                                frame 4 {
                                n145 = local read "RAM"() -> (w728:bool)
                                n146 = Select(t="*G18", s=w728, f="*R18") -> (s? t:f=w725:string)
                                }
                                frame 5 {
                                n147 = local read "RAM"() -> (w732:bool)
                                n148 = Select(t="*G19", s=w732, f="*R19") -> (s? t:f=w729:string)
                                }
                              }
                            }
                            frame #1 {
                              n149 = Unbundle(w736) -> ("VISA resource name out"=w741:refnum<visa-resource-name>, "error out"=w739:errorcluster, "Delay (ms)"=w740:u32, "Write/\nRead"=w738:bool)
                              n150 = call "I3252_Comm_Interface.vi"("VISA resource name in"=w741, "error in"=w739, "Delay (ms)"=w740, "Write"=w738, "String to Write"=w737, "Read"=w738) -> ("VISA resource name out"=w734:refnum<visa-resource-name>, "error out"=w735:errorcluster, "Read String"=w733:string)  [unwired: 2 in]
                            }
                            frame #2 {
                              n151 = case shown="5" w742 {
                                tunnel: w743 -> [_ w747 w751 w755]
                                frame 0, Default {
                                }
                                frame 3 {
                                n152 = String Subset(string=w747, offset (0)=3) -> (substring=w745:string)  [unwired: 1 in]
                                n153 = Hexadecimal String To Number(string=w745) -> (number=→"P (PB1) Istwert":u32)  [unwired: 2 in, 1 out]
                                }
                                frame 4 {
                                n154 = String Subset(string=w751, offset (0)=3) -> (substring=w749:string)  [unwired: 1 in]
                                n155 = Hexadecimal String To Number(string=w749) -> (number=→"I ( Reset1) Istwert":u32)  [unwired: 2 in, 1 out]
                                }
                                frame 5 {
                                n156 = String Subset(string=w755, offset (0)=3) -> (substring=w753:string)  [unwired: 1 in]
                                n157 = Hexadecimal String To Number(string=w753) -> (number=→"D (Rate) IstWert":u32)  [unwired: 2 in, 1 out]
                                }
                              }
                            }
                          }
                        }
                      }
                      frame #2 {
                        n158 = property on="Set PID" class="Bool"("Blinking"=FALSE) -> ()  [unwired: 2 in, 2 out]
                      }
                    }
                    n159 = Not(x="Set PID") -> (.not. x?=w682:bool)
                  }
                  event "Get Values": Value Change {
                    n160 = event-data() -> ()  [unwired: 1 in, 1 out]
                    n161 = stacked-sequence {
                      tunnel: w759 -> [_ w766 _]
                      tunnel: [_ w765 _] -> w758
                      tunnel: [_ w764 _] -> w757
                      frame #0 {
                        n162 = property on="Get Values" class="Bool"("Blinking"=TRUE) -> ()  [unwired: 2 in, 2 out]
                        n163 = property on="ON" class="Bool (strict)"("Blinking"=FALSE) -> ()  [unwired: 2 in, 2 out]
                      }
                      frame #1 {
                        n164 = for {
                          N: 6 -> [_]
                          tunnel: w766 -> [w770]
                          tunnel: [w769] -> w765
                          tunnel: [w768] -> w764
                          i -> [w772]
                          n165 = flat-sequence {
                            tunnel: w772 -> [w774]
                            tunnel: [w775] -> w771
                            tunnel: w771 -> [w797]
                            tunnel: [w798] -> w773
                            tunnel: w770 -> [w796]
                            tunnel: [w795] -> w768
                            tunnel: [w794] -> w769
                            tunnel: w773 -> [w804]
                            tunnel: w772 -> [w803]
                            frame #0 {
                              n166 = case shown="0, Default" w774 {
                                tunnel: [w778 w782 w786 "*R27" "*R28" w792] -> w775
                                frame 0, Default {
                                n167 = local read "RAM"() -> (w779:bool)
                                n168 = Select(t="*G17", s=w779, f="*R17") -> (s? t:f=w778:string)
                                }
                                frame 1 {
                                n169 = local read "RAM"() -> (w783:bool)
                                n170 = Select(t="*G18", s=w783, f="*R18") -> (s? t:f=w782:string)
                                }
                                frame 2 {
                                n171 = local read "RAM"() -> (w787:bool)
                                n172 = Select(t="*G19", s=w787, f="*R19") -> (s? t:f=w786:string)
                                }
                                frame 3 {
                                }
                                frame 4 {
                                }
                                frame 5 {
                                n173 = local read "RAM"() -> (w793:bool)
                                n174 = Select(t="*G01", s=w793, f="*R01") -> (s? t:f=w792:string)
                                }
                              }
                            }
                            frame #1 {
                              n175 = Unbundle(w796) -> ("VISA resource name out"=w802:refnum<visa-resource-name>, "error out"=w800:errorcluster, "Delay (ms)"=w801:u32, "Write/\nRead"=w799:bool)
                              n176 = call "I3252_Comm_Interface.vi"("VISA resource name in"=w802, "error in"=w800, "Delay (ms)"=w801, "Write"=w799, "String to Write"=w797, "Read"=w799) -> ("VISA resource name out"=w794:refnum<visa-resource-name>, "error out"=w795:errorcluster, "Read String"=w798:string)  [unwired: 2 in]
                            }
                            frame #2 {
                              n177 = case shown="0, Default" w803 {
                                tunnel: w804 -> [w806 w810 w814 w818 w822 w826]
                                frame 0, Default {
                                n178 = String Subset(string=w806, offset (0)=3) -> (substring=w807:string)  [unwired: 1 in]
                                n179 = Hexadecimal String To Number(string=w807) -> (number=w805:u32)  [unwired: 2 in, 1 out]
                                n180 = local write "P (PB1) Sollwert"(w805) -> ()
                                n181 = local write "P (PB1) Istwert"(w805) -> ()
                                }
                                frame 1 {
                                n182 = String Subset(string=w810, offset (0)=3) -> (substring=w811:string)  [unwired: 1 in]
                                n183 = Hexadecimal String To Number(string=w811) -> (number=w809:u32)  [unwired: 2 in, 1 out]
                                n184 = local write "I ( Reset1) Sollwert"(w809) -> ()
                                n185 = local write "I ( Reset1) Istwert"(w809) -> ()
                                }
                                frame 2 {
                                n186 = String Subset(string=w814, offset (0)=3) -> (substring=w815:string)  [unwired: 1 in]
                                n187 = Hexadecimal String To Number(string=w815) -> (number=w813:u32)  [unwired: 2 in, 1 out]
                                n188 = local write "D (Rate) Sollwert"(w813) -> ()
                                n189 = local write "D (Rate) IstWert"(w813) -> ()
                                }
                                frame 3 {
                                n190 = String Subset(string=w818, offset (0)=3) -> (substring=w819:string)  [unwired: 1 in]
                                n191 = Hexadecimal String To Number(string=w819) -> (number=w817:u32)  [unwired: 2 in, 1 out]
                                n192 = local write "% LOW Istwert"(w817) -> ()
                                n193 = local write "% LOW Sollwert"(w817) -> ()
                                }
                                frame 4 {
                                n194 = String Subset(string=w822, offset (0)=3) -> (substring=w823:string)  [unwired: 1 in]
                                n195 = Hexadecimal String To Number(string=w823) -> (number=w821:u32)  [unwired: 2 in, 1 out]
                                n196 = local write "% High Sollwert"(w821) -> ()
                                n197 = local write "% HIGH Istwert"(w821) -> ()
                                }
                                frame 5 {
                                n198 = call "I3252_Edit_Setpoint.vi"("Read String"=w826) -> ("Setpoint is"=w825:dbl)
                                n199 = local write "SP 1 is (°C)"(w825) -> ()
                                }
                              }
                            }
                          }
                        }
                      }
                      frame #2 {
                        n200 = property on="Get Values" class="Bool"("Blinking"=FALSE) -> ()  [unwired: 2 in, 2 out]
                      }
                    }
                    n201 = Not(x="Get Values") -> (.not. x?=w761:bool)
                  }
                  event "RAM": Value Change {
                    n202 = event-data() -> ()  [unwired: 1 in, 1 out]
                    n203 = stacked-sequence {
                      tunnel: w830 -> [_ w837 _]
                      tunnel: [_ w836 _] -> w829
                      tunnel: [_ w835 _] -> w828
                      frame #0 {
                        n204 = property on="RAM" class="Bool (strict)"("Blinking"=TRUE) -> ()  [unwired: 2 in, 2 out]
                        n205 = property on="ON" class="Bool (strict)"("Blinking"=FALSE) -> ()  [unwired: 2 in, 2 out]
                      }
                      frame #1 {
                        n206 = for {
                          N: 6 -> [_]
                          tunnel: w837 -> [w841]
                          tunnel: [w840] -> w836
                          tunnel: [w839] -> w835
                          i -> [w843]
                          n207 = flat-sequence {
                            tunnel: w843 -> [w845]
                            tunnel: [w846] -> w842
                            tunnel: w842 -> [w865]
                            tunnel: [w866] -> w844
                            tunnel: w841 -> [w869]
                            tunnel: [w868] -> w839
                            tunnel: [w867] -> w840
                            tunnel: w844 -> [w875]
                            tunnel: w843 -> [w874]
                            frame #0 {
                              n208 = case shown="0, Default" w845 {
                                tunnel: [w849 w853 w857 "*R27" "*R28" w863] -> w846
                                frame 0, Default {
                                n209 = local read "RAM"() -> (w850:bool)
                                n210 = Select(t="*G17", s=w850, f="*R17") -> (s? t:f=w849:string)
                                }
                                frame 1 {
                                n211 = local read "RAM"() -> (w854:bool)
                                n212 = Select(t="*G18", s=w854, f="*R18") -> (s? t:f=w853:string)
                                }
                                frame 2 {
                                n213 = local read "RAM"() -> (w858:bool)
                                n214 = Select(t="*G19", s=w858, f="*R19") -> (s? t:f=w857:string)
                                }
                                frame 3 {
                                }
                                frame 4 {
                                }
                                frame 5 {
                                n215 = local read "RAM"() -> (w864:bool)
                                n216 = Select(t="*G01", s=w864, f="*R01") -> (s? t:f=w863:string)
                                }
                              }
                            }
                            frame #1 {
                              n217 = Unbundle(w869) -> ("VISA resource name out"=w873:refnum<visa-resource-name>, "error out"=w871:errorcluster, "Delay (ms)"=w872:u32, "Write/\nRead"=w870:bool)
                              n218 = call "I3252_Comm_Interface.vi"("VISA resource name in"=w873, "error in"=w871, "Delay (ms)"=w872, "Write"=w870, "String to Write"=w865, "Read"=w870) -> ("VISA resource name out"=w867:refnum<visa-resource-name>, "error out"=w868:errorcluster, "Read String"=w866:string)  [unwired: 2 in]
                            }
                            frame #2 {
                              n219 = case shown="0, Default" w874 {
                                tunnel: w875 -> [w877 w881 w885 w889 w893 w897]
                                frame 0, Default {
                                n220 = String Subset(string=w877, offset (0)=3) -> (substring=w878:string)  [unwired: 1 in]
                                n221 = Hexadecimal String To Number(string=w878) -> (number=w876:u32)  [unwired: 2 in, 1 out]
                                n222 = local write "P (PB1) Sollwert"(w876) -> ()
                                n223 = local write "P (PB1) Istwert"(w876) -> ()
                                }
                                frame 1 {
                                n224 = String Subset(string=w881, offset (0)=3) -> (substring=w882:string)  [unwired: 1 in]
                                n225 = Hexadecimal String To Number(string=w882) -> (number=w880:u32)  [unwired: 2 in, 1 out]
                                n226 = local write "I ( Reset1) Sollwert"(w880) -> ()
                                n227 = local write "I ( Reset1) Istwert"(w880) -> ()
                                }
                                frame 2 {
                                n228 = String Subset(string=w885, offset (0)=3) -> (substring=w886:string)  [unwired: 1 in]
                                n229 = Hexadecimal String To Number(string=w886) -> (number=w884:u32)  [unwired: 2 in, 1 out]
                                n230 = local write "D (Rate) IstWert"(w884) -> ()
                                n231 = local write "D (Rate) Sollwert"(w884) -> ()
                                }
                                frame 3 {
                                n232 = String Subset(string=w889, offset (0)=3) -> (substring=w890:string)  [unwired: 1 in]
                                n233 = Hexadecimal String To Number(string=w890) -> (number=w888:u32)  [unwired: 2 in, 1 out]
                                n234 = local write "% LOW Istwert"(w888) -> ()
                                n235 = local write "% LOW Sollwert"(w888) -> ()
                                }
                                frame 4 {
                                n236 = String Subset(string=w893, offset (0)=3) -> (substring=w894:string)  [unwired: 1 in]
                                n237 = Hexadecimal String To Number(string=w894) -> (number=w892:u32)  [unwired: 2 in, 1 out]
                                n238 = local write "% HIGH Istwert"(w892) -> ()
                                n239 = local write "% High Sollwert"(w892) -> ()
                                }
                                frame 5 {
                                n240 = call "I3252_Edit_Setpoint.vi"("Read String"=w897) -> ("Setpoint is"=w896:dbl)
                                n241 = local write "SP 1 is (°C)"(w896) -> ()
                                }
                              }
                            }
                          }
                        }
                      }
                      frame #2 {
                        n242 = property on="RAM" class="Bool (strict)"("Blinking"=FALSE) -> ()  [unwired: 2 in, 2 out]
                      }
                    }
                    n243 = Not(x="RAM") -> (.not. x?=w832:bool)
                  }
                  event "Set Gauge to Zero": Value Change {
                    n244 = event-data() -> ()  [unwired: 1 in, 1 out]
                    n245 = flat-sequence {
                      tunnel: w903 -> [w908]
                      tunnel: [w908] -> w902
                      tunnel: w902 -> [w910]
                      tunnel: [w914] -> w901
                      tunnel: [w913] -> w900
                      tunnel: [w910] -> w899
                      tunnel: w901 -> [w920]
                      tunnel: w900 -> [w919]
                      tunnel: w899 -> [w915]
                      frame #0 {
                        n246 = property on="Set Gauge to Zero" class="Bool"("Blinking"=TRUE) -> ()  [unwired: 2 in, 2 out]
                      }
                      frame #1 {
                        w911 = 0 items=["sensor 1", "sensor 2", "test"] ("Sensor Nr.:")
                        n247 = call "DUAL GAUGE-Get Pressure,Status.vi"("Sensor Nr.:"=w911, "Referenz in"=w910) -> ("Pressure"=w914:dbl)  [unwired: 6 in, 3 out]
                        n248 = call "DUAL GAUGE-Offset display.vi"("W/R"=FALSE, "Referenz in"=w910) -> ("Sensor 1 Get"=w913:dbl)  [unwired: 6 in, 3 out]
                      }
                      frame #2 {
                        n249 = Add(x=w920, y=w919) -> (x+y=w916:dbl)
                        n250 = call "DUAL GAUGE-Offset display.vi"("W/R"=TRUE, "Sensor 1 Set"=w916, "Referenz in"=w915) -> ("Sensor 1 Get"=→"Current Offset (mbar)":dbl)  [unwired: 5 in, 3 out]
                      }
                      frame #3 {
                        n251 = property on="Set Gauge to Zero" class="Bool"("Blinking"=TRUE) -> ()  [unwired: 2 in, 2 out]
                      }
                    }
                    n252 = Unbundle(w907) -> ("VISA resource name out"=w906:refnum<visa-resource-name>, "error out"=w905:errorcluster)  [unwired: 2 out]
                  }
                  event "Write to File": Value Change {
                    n253 = event-data() -> ("NewVal"=w926:bool)  [unwired: 1 in]
                    n254 = local read "File Path"() -> (w922:path)
                    n255 = case shown="True" w926 {
                      tunnel: w922 -> [_ w934]
                      tunnel: "User" -> [_ w933]
                      tunnel: "Sample" -> [_ w932]
                      tunnel: [path "" ("File Path") w931] -> w923
                      frame False {
                      }
                      frame True {
                        n256 = call "Header.vi"("Sample"=w932, "User"=w933, "File Path"=w934) -> ("File Path"=w931:path)
                      }
                    }
                    n257 = Unbundle(w929) -> ("VISA resource name out"=w928:refnum<visa-resource-name>, "error out"=w927:errorcluster)  [unwired: 2 out]
                    n258 = local write "File Path"(w923) -> ()
                  }
                  event "Ramp": Value Change {
                    n259 = event-data() -> ()  [unwired: 1 in, 6 out]
                    n260 = stacked-sequence {
                      tunnel: [_ w942 _ _] -> w935
                      tunnel: [_ w941 _ _] -> w936
                      tunnel: w937 -> [_ w940 w991 _]
                      frame #0 {
                        n261 = property on="Ramp" class="Bool (strict)"("Blinking"=TRUE) -> ()  [unwired: 2 in, 2 out]
                      }
                      frame #1 {
                        n262 = for {
                          N: 6 -> [_]
                          tunnel: [w948] -> w942
                          tunnel: [w947] -> w941
                          tunnel: w940 -> [w946]
                          i -> [w944]
                          n263 = flat-sequence {
                            tunnel: w944 -> [w950]
                            tunnel: [w949] -> w945
                            tunnel: [w983] -> w948
                            tunnel: [w984] -> w947
                            tunnel: w946 -> [w985]
                            tunnel: w945 -> [w982]
                            frame #0 {
                              n264 = case shown="5" w950 {
                                tunnel: ["*D03" w954 w956 w968 "*E03" ("string") "*Z02" ("string")] -> w949
                                frame 0, Default {
                                }
                                frame 1 {
                                n265 = local read "Ramp"() -> (w952:bool)
                                n266 = Select(t="*W0D78", s=w952, f="*W0D60") -> (s? t:f=w954:string)
                                }
                                frame 2 {
                                n267 = local read "Ramp"() -> (w957:bool)
                                n268 = case shown="True" w957 {
                                tunnel: ["*W0E0000" ("string") w959] -> w956
                                frame False {
                                }
                                frame True {
                                n269 = Multiply(x="Hours", y=100.0) -> (x*y=w965:dbl)
                                n270 = Add(x=w965, y="Minutes") -> (x+y=w962:dbl)
                                n271 = Number To Hexadecimal String(1:i16 4 ("width (-)"), 2:w962) -> (0:w963:string)
                                n272 = Concatenate Strings("*W0E" ("string"), w963) -> (w959:string)
                                }
                                }
                                }
                                frame 3 {
                                n273 = local read "Ramp"() -> (w969:bool)
                                n274 = case shown="True" w969 {
                                tunnel: ["*W1E0000" ("string") w971] -> w968
                                frame False {
                                }
                                frame True {
                                n275 = Multiply(x="Soak Hours", y=100.0) -> (x*y=w977:dbl)
                                n276 = Add(x=w977, y="Soak Minutes") -> (x+y=w974:dbl)
                                n277 = Number To Hexadecimal String(1:i16 4 ("width (-)"), 2:w974) -> (0:w975:string)
                                n278 = Concatenate Strings("*W1E" ("string"), w975) -> (w971:string)
                                }
                                }
                                }
                                frame 4 {
                                }
                                frame 5 {
                                }
                              }
                            }
                            frame #1 {
                              n279 = Unbundle(w985) -> ("VISA resource name out"=w986:refnum<visa-resource-name>, "error out"=w988:errorcluster, "Delay (ms)"=w987:u32, "Write/\nRead"=w989:bool)
                              n280 = call "I3252_Comm_Interface.vi"("VISA resource name in"=w986, "error in"=w988, "Delay (ms)"=w987, "Write"=w989, "String to Write"=w982, "Read"=w989) -> ("VISA resource name out"=w984:refnum<visa-resource-name>, "error out"=w983:errorcluster)  [unwired: 2 in, 1 out]
                            }
                          }
                          n281 = Wait (ms)(milliseconds to wait=u32 1000) -> ()  [unwired: 1 out]
                        }
                      }
                      frame #2 {
                        n282 = local read "Ramp"() -> (w990:bool)
                        n283 = case shown="True" w990 {
                          tunnel: w991 -> [_ w992]
                          frame False {
                          }
                          frame True {
                            n284 = Multiply(x=10.0, y="Setpoint") -> (x*y=w997:dbl)
                            n285 = Number To Hexadecimal String(1:i16 5 ("width (-)"), 2:w997) -> (0:w998:string)
                            n286 = Concatenate Strings("*P012", w998) -> (w994:string)
                            n287 = Wait (ms)(milliseconds to wait=u32 4000) -> ()  [unwired: 1 out]
                            n288 = Unbundle(w992) -> ("VISA resource name out"=w1000:refnum<visa-resource-name>, "error out"=w1002:errorcluster, "Delay (ms)"=w1001:u32, "Write/\nRead"=w1003:bool)
                            n289 = call "I3252_Comm_Interface.vi"("VISA resource name in"=w1000, "error in"=w1002, "Delay (ms)"=w1001, "Write"=w1003, "String to Write"=w994, "Read"=w1003) -> ()  [unwired: 2 in, 3 out]
                          }
                        }
                      }
                      frame #3 {
                        n290 = property on="Ramp" class="Bool (strict)"("Blinking"=FALSE) -> ()  [unwired: 2 in, 2 out]
                      }
                    }
                  }
                  event "Get SetPoint": Value Change {
                    n291 = event-data() -> ()  [unwired: 1 in, 6 out]
                    n292 = Unbundle(w1009) -> ("VISA resource name out"=w1013:refnum<visa-resource-name>, "error out"=w1015:errorcluster, "Delay (ms)"=w1014:u32, "Write/\nRead"=w1016:bool)
                    n293 = call "I3252_Comm_Interface.vi"("VISA resource name in"=w1013, "error in"=w1015, "Delay (ms)"=w1014, "Write"=w1016, "String to Write"="*G01", "Read"=w1016) -> ("VISA resource name out"=w1008:refnum<visa-resource-name>, "error out"=w1007:errorcluster, "Read String"=w1012:string)  [unwired: 2 in]
                    n294 = call "I3252_Edit_Setpoint.vi"("Read String"=w1012) -> ("Setpoint is"=→"Get Actual Set Point":dbl)
                  }
                  event "Emissivity\n(eg: 0500)": Value Change {
                    n295 = event-data() -> ()  [unwired: 1 in, 6 out]
                    n296 = Concatenate Strings("em" ("string"), "Emissivity\n(eg: 0500)", "\\n" ("string")) -> (w1020:string)
                    n297 = VISA Write(VISA resource name=w1021, write buffer=w1020) -> ()  [unwired: 1 in, 3 out]
                  }
                }
              }
              n298 = Bundle(cluster=w427, "VISA resource name out"=w426, "error out"=w425) -> (w424:T7)  [unwired: 2 in]
            }
            frame #2 {
            }
            frame #3 {
              (unwired) "Daniel Schuster (geb. 20.03.1988)"
              n299 = node-c288(w1083) -> (w1092:T3)  [unwired: 2 in]
              n300 = node-c288(w1098) -> (w1101:T3)  [unwired: 2 in]
              n301 = node-c288(w1088) -> (w1090:T3)  [unwired: 2 in]
              n302 = node-c288(w1097) -> (w1105:T3)  [unwired: 2 in]
              n303 = timed-sequence {
                timing: w1092 -> [_]
                timing-out: [_] -> w1091
                tunnel: w1067 -> [w1175]
                tunnel: w1066 -> [w1171]
                tunnel: [w1174] -> w1059
                tunnel: w1058 -> [w1173]
                tunnel: w1057 -> [w1172]
                tunnel: [w1170] -> w1056
                tunnel: [w1169] -> w1055
                tunnel: [w1168] -> w1053
                n304 = timed-flat-sequence {
                  tunnel: w1175 -> [w1184]
                  tunnel: [w1183] -> w1174
                  tunnel: w1173 -> [w1182]
                  tunnel: w1172 -> [w1181]
                  tunnel: w1171 -> [w1180]
                  tunnel: [w1178] -> w1170
                  tunnel: [w1177] -> w1169
                  tunnel: [w1176] -> w1168
                  n305 = node-c288() -> ()  [unwired: 1 in, 1 out]
                  n306 = case shown="False" "ON (TPG 2)" {
                    tunnel: w1180 -> [w1189 w1195]
                    tunnel: w1181 -> [w1188 w1194]
                    tunnel: [w1187 w1193] -> w1177
                    tunnel: [w1186 w1192] -> w1176
                    frame False {
                      w1190 = 0.0 ("Pressure")
                      n307 = property on="ON (TPG 2)" class="Bool (strict)"("Blinking"=FALSE) -> ()  [unwired: 2 in, 2 out]
                      n308 = Bundle("Pressure"=w1190, "Pressure"=w1190) -> (w1187:cluster{"Pressure":dbl, "Pressure":dbl})  [unwired: 1 in]
                      n309 = Bundle("TPG 2 COM"=w1189, "error out"=w1188) -> (w1186:T8)  [unwired: 1 in]
                    }
                    frame True {
                      n310 = stacked-sequence {
                        tunnel: w1195 -> [_ w1208]
                        tunnel: [_ w1204] -> w1193
                        tunnel: [_ w1200] -> w1192
                        tunnel: w1194 -> [_ w1197]
                        frame #0 {
                          n311 = property on="ON (TPG 2)" class="Bool (strict)"("Blinking"=TRUE) -> ()  [unwired: 2 in, 2 out]
                        }
                        frame #1 {
                          n312 = call "PresureGetSubVI.vi"("COM in"=w1208, "Fehler (Eingang)"=w1197) -> ("Status Gauge#1"=→"Status Gauge 2#1":i32, "Status Gauge#2"=→"Status Gauge 2#2":i32, "COM out"=w1201:refnum<visa-resource-name>, "Pressure Gauge#1"=w1202:dbl, "Pressure Gauge#2"=w1205:dbl, "Cluster (Ausgang)"=w1198:errorcluster)  [unwired: 12 in]
                          "Pressure Gauge 2#1" <- w1202
                          "Pressure Gauge 2#2" <- w1205
                          n313 = Bundle("COM out"=w1201, "Cluster (Ausgang)"=w1198) -> (w1200:T9)  [unwired: 1 in]
                          n314 = Unbundle(w1198) -> ("status"=w1199:bool, "code"=w1203:i32)  [unwired: 1 out]
                          n315 = Bundle("status"=w1199, "code"=w1203) -> ()  [unwired: 1 in, 1 out]
                          n316 = Bundle("Pressure Gauge#1"=w1202, "Pressure Gauge#2"=w1205) -> (w1204:T10)  [unwired: 1 in]
                        }
                      }
                    }
                  }
                  n317 = case shown="False" "ON (TPG 1)" {
                    tunnel: w1184 -> [w1212 w1218]
                    tunnel: [w1211 w1217] -> w1183
                    tunnel: w1182 -> [w1210 w1216]
                    tunnel: [w1209 w1215] -> w1178
                    frame False {
                      w1213 = 0.0 ("Pressure")
                      n318 = property on="ON (TPG 1)" class="Bool (strict)"("Blinking"=FALSE) -> ()  [unwired: 2 in, 2 out]
                      n319 = Bundle("Pressure"=w1213, "Pressure"=w1213) -> (w1209:cluster{"Pressure":dbl, "Pressure":dbl})  [unwired: 1 in]
                      n320 = Bundle("TPG 1 COM"=w1212, "error out"=w1210) -> (w1211:T11)  [unwired: 1 in]
                    }
                    frame True {
                      n321 = stacked-sequence {
                        tunnel: w1218 -> [_ w1231]
                        tunnel: [_ w1224] -> w1217
                        tunnel: w1216 -> [_ w1221]
                        tunnel: [_ w1220] -> w1215
                        frame #0 {
                          n322 = property on="ON (TPG 1)" class="Bool (strict)"("Blinking"=TRUE) -> ()  [unwired: 2 in, 2 out]
                        }
                        frame #1 {
                          n323 = call "PresureGetSubVI.vi"("COM in"=w1231, "Fehler (Eingang)"=w1221) -> ("Status Gauge#1"=→"Status Gauge 1#1":i32, "Status Gauge#2"=→"Status Gauge 1#2":i32, "COM out"=w1225:refnum<visa-resource-name>, "Pressure Gauge#1"=w1226:dbl, "Pressure Gauge#2"=w1228:dbl, "Cluster (Ausgang)"=w1222:errorcluster)  [unwired: 12 in]
                          "Pressure Gauge 1#1" <- w1226
                          "Pressure Gauge 1#2" <- w1228
                          n324 = Bundle("COM out"=w1225, "Cluster (Ausgang)"=w1222) -> (w1224:T9)  [unwired: 1 in]
                          n325 = Unbundle(w1222) -> ("status"=w1223:bool, "code"=w1227:i32)  [unwired: 1 out]
                          n326 = Bundle("status"=w1223, "code"=w1227) -> ()  [unwired: 1 in, 1 out]
                          n327 = Bundle("Pressure Gauge#1"=w1226, "Pressure Gauge#2"=w1228) -> (w1220:T10)  [unwired: 1 in]
                        }
                      }
                    }
                  }
                  n328 = node-c288() -> ()  [unwired: 1 in, 1 out]
                }
              }
              n329 = case shown="True" "Pyrometer" {
                tunnel: [0 w1111] -> w1051
                tunnel: w1049 -> [w1107 w1110]
                tunnel: w1048 -> [_ w1109]
                tunnel: [w1107 w1108] -> w1047
                frame False {
                }
                frame True {
                  n330 = flat-sequence {
                    tunnel: [w1120] -> w1115
                    tunnel: [w1119] -> w1114
                    tunnel: w1110 -> [w1118]
                    tunnel: w1109 -> [w1116]
                    tunnel: w1115 -> [w1123]
                    tunnel: w1114 -> [w1122]
                    tunnel: [w1123] -> w1113
                    tunnel: [w1122] -> w1112
                    tunnel: w1113 -> [w1130]
                    tunnel: w1112 -> [w1129]
                    tunnel: [w1127] -> _
                    tunnel: [w1124] -> w1111
                    tunnel: [w1126] -> w1108
                    frame #0 {
                      n331 = VISA Write(VISA resource name=w1118, write buffer="00ms\n" ("string"), error in (no error)=w1116) -> (VISA resource name out=w1120:refnum<visa-resource-name>, error out=w1119:errorcluster)  [unwired: 1 out]
                    }
                    frame #1 {
                      n332 = Wait (ms)(milliseconds to wait=u32 500 ("wait")) -> ()  [unwired: 1 out]
                    }
                    frame #2 {
                      n333 = property class="Instr"(reference=w1130, error in=w1129) -> (reference out=w1131:refnum<visa-resource-name>, error out=w1128:errorcluster, "Bytes at Port"=w1132:u32)
                      n334 = VISA Read(VISA resource name=w1131, byte count=w1132, error in (no error)=w1128) -> (VISA resource name out=w1126:refnum<visa-resource-name>, read buffer=w1125:string, error out=w1127:errorcluster)  [unwired: 1 out]
                      n335 = Fract/Exp String To Number(string=w1125) -> (number=w1124:dbl)  [unwired: 3 in, 1 out]
                      "Pyro Temp" <- w1124
                    }
                  }
                }
              }
              n336 = timed-sequence {
                timing: w1101 -> [_]
                timing-out: [_] -> w1100
                tunnel: w1099 -> [w1241]
                tunnel: [w1240] -> w1094
                tunnel: [w1239] -> w1093
                tunnel: [w1238] -> w1080
                n337 = timed-flat-sequence {
                  tunnel: w1241 -> [w1245]
                  tunnel: [w1244] -> w1240
                  tunnel: [w1243] -> w1239
                  tunnel: [w1242] -> w1238
                  n338 = node-c288() -> ()  [unwired: 1 in, 1 out]
                  n339 = case shown="False" "ON" {
                    tunnel: w1245 -> [w1249 w1254]
                    tunnel: [w1248 w1253] -> w1244
                    tunnel: [w1247 w1252] -> w1243
                    tunnel: [_ w1251] -> w1242
                    frame False {
                      n340 = Unbundle(w1249) -> ("VISA resource name out"=w1248:refnum<visa-resource-name>, "error out"=w1247:errorcluster)  [unwired: 2 out]
                      n341 = property on="ON" class="Bool (strict)"("Blinking"=FALSE) -> ()  [unwired: 2 in, 2 out]
                    }
                    frame True {
                      n342 = stacked-sequence {
                        tunnel: w1254 -> [_ w1259]
                        tunnel: [_ w1258] -> w1253
                        tunnel: [_ w1257] -> w1252
                        tunnel: [_ w1256] -> w1251
                        frame #0 {
                          n343 = property on="ON" class="Bool (strict)"("Blinking"=TRUE) -> ()  [unwired: 2 in, 2 out]
                        }
                        frame #1 {
                          n344 = Unbundle(w1259) -> ("VISA resource name out"=w1263:refnum<visa-resource-name>, "error out"=w1261:errorcluster, "Delay (ms)"=w1262:u32, "Write/\nRead"=w1260:bool)
                          n345 = call "I3252_Comm_Interface.vi"("VISA resource name in"=w1263, "error in"=w1261, "Delay (ms)"=w1262, "Write"=w1260, "String to Write"="*V01", "Read"=w1260) -> ("VISA resource name out"=w1258:refnum<visa-resource-name>, "error out"=w1257:errorcluster, "Read String"=w1256:string)  [unwired: 2 in]
                        }
                      }
                    }
                  }
                  n346 = node-c288() -> ()  [unwired: 1 in, 1 out]
                }
              }
              n347 = timed-sequence {
                timing: w1090 -> [_]
                timing-out: [_] -> w1089
                tunnel: w1087 -> [w1137]
                tunnel: w1086 -> [w1136]
                tunnel: [w1135] -> w1084
                tunnel: [w1134] -> w1085
                tunnel: [w1133] -> w1081
                n348 = timed-flat-sequence {
                  tunnel: w1137 -> [w1142]
                  tunnel: w1136 -> [w1141]
                  tunnel: [w1140] -> w1135
                  tunnel: [w1139] -> w1134
                  tunnel: [w1138] -> w1133
                  n349 = node-c288() -> ()  [unwired: 1 in, 1 out]
                  n350 = case shown="False" "ON" {
                    tunnel: w1142 -> [w1146 w1152]
                    tunnel: w1141 -> [w1147 w1151]
                    tunnel: [w1146 w1150] -> w1140
                    tunnel: [w1147 w1149] -> w1139
                    tunnel: [0.0 ("Reading") w1148] -> w1138
                    frame False {
                      n351 = property on="ON" class="Bool (strict)"("Blinking"=FALSE) -> ()  [unwired: 2 in, 2 out]
                    }
                    frame True {
                      n352 = stacked-sequence {
                        tunnel: w1152 -> [_ w1159]
                        tunnel: w1151 -> [_ w1158]
                        tunnel: [_ w1157] -> w1150
                        tunnel: [_ w1156] -> w1149
                        tunnel: [_ w1154] -> w1148
                        frame #0 {
                          n353 = property on="ON" class="Bool (strict)"("Blinking"=TRUE) -> ()  [unwired: 2 in, 2 out]
                        }
                        frame #1 {
                          n354 = call "VC840_Read.vi"("error in (no error)"=w1158, "VISA resource name"=w1159) -> ("error out"=w1156:errorcluster, "Unit"=→"Unit 2":string, "Reading"=w1154:dbl, "VISA resource name out"=w1157:refnum<visa-resource-name>, "Status"=→"Status 2":T2, "Mode"=→"Mode 2":enum16{"?", "Diode", "Beep", "DC", "AC"})  [unwired: 4 out]
                          "Reading 2" <- w1154
                        }
                      }
                    }
                  }
                  n355 = node-c288() -> ()  [unwired: 1 in, 1 out]
                }
              }
              n356 = timed-sequence {
                timing: w1105 -> [_]
                timing-out: [_] -> w1104
                tunnel: w1103 -> [w1275]
                tunnel: w1102 -> [w1274]
                tunnel: [w1273] -> w1096
                tunnel: [w1272] -> w1095
                tunnel: [w1271] -> w1082
                n357 = timed-flat-sequence {
                  tunnel: w1275 -> [w1280]
                  tunnel: w1274 -> [w1279]
                  tunnel: [w1278] -> w1273
                  tunnel: [w1277] -> w1272
                  tunnel: [w1276] -> w1271
                  n358 = node-c288() -> ()  [unwired: 1 in, 1 out]
                  n359 = case shown="False" "ON" {
                    tunnel: w1280 -> [w1284 w1290]
                    tunnel: w1279 -> [w1285 w1289]
                    tunnel: [w1284 w1288] -> w1278
                    tunnel: [w1285 w1287] -> w1277
                    tunnel: [0.0 ("Reading") w1286] -> w1276
                    frame False {
                      n360 = property on="ON" class="Bool (strict)"("Blinking"=FALSE) -> ()  [unwired: 2 in, 2 out]
                    }
                    frame True {
                      n361 = stacked-sequence {
                        tunnel: w1290 -> [_ w1297]
                        tunnel: w1289 -> [_ w1296]
                        tunnel: [_ w1295] -> w1288
                        tunnel: [_ w1294] -> w1287
                        tunnel: [_ w1292] -> w1286
                        frame #0 {
                          n362 = property on="ON" class="Bool (strict)"("Blinking"=TRUE) -> ()  [unwired: 2 in, 2 out]
                        }
                        frame #1 {
                          n363 = call "VC840_Read.vi"("error in (no error)"=w1296, "VISA resource name"=w1297) -> ("error out"=w1294:errorcluster, "Unit"=→"Unit 1":string, "Reading"=w1292:dbl, "VISA resource name out"=w1295:refnum<visa-resource-name>, "Status"=→"Status 1":T2, "Mode"=→"Mode 1":enum16{"?", "Diode", "Beep", "DC", "AC"})  [unwired: 4 out]
                          "Reading 1" <- w1292
                        }
                      }
                    }
                  }
                  n364 = node-c288() -> ()  [unwired: 1 in, 1 out]
                }
              }
              n365 = Tick Count (ms)() -> (millisecond timer value=w1068:u32)
              n366 = Subtract(x=w1068, y=w1073) -> (x-y=w1072:u32)
              n367 = Divide(x=w1072, y=u32 1000) -> (x/y=w1070:dbl)
              n368 = node-c288(w1104) -> ()  [unwired: 1 out]
              n369 = node-c288(w1089) -> ()  [unwired: 1 out]
              n370 = node-c288(w1100) -> ()  [unwired: 1 out]
              n371 = To Double Precision Float(number=w1070) -> (double precision float=w1074:dbl)
              "current time (s)" <- w1074
              n372 = node-c288(w1091) -> ()  [unwired: 1 out]
              n373 = Unbundle(w1055) -> ("Pressure Gauge#1"=w1054:dbl, "Pressure Gauge#2"=w1052:dbl)
              "Pressure OpenPort2" <- w1052
              "Pressure Pirani 2" <- w1054
              n374 = Unbundle(w1056) -> ("Pressure Gauge#1"=w1065:dbl, "Pressure Gauge#2"=w1060:dbl)
              "Pressure Baratron 2" <- w1065
              "Pressure FullRange 2" <- w1060
            }
            frame #4 {
              n375 = Build Array (concatenate)(w1319, w1323) -> (w1318:dbl[])
              n376 = Build Array (concatenate)(w1322, w1324) -> (w1317:dbl[])
              n377 = Build Array (concatenate)(w1320, w1311) -> (w1315:dbl[])
              n378 = Build Array (concatenate)(w1321, w1312) -> (w1316:dbl[])
              n379 = Greater?(x=w1343, y="Pressure Limit (mbar)") -> (0:w1346:bool)
              n380 = case shown="False" w1346 {
                frame False {
                  n381 = property on="Standby" class="Bool (strict)"("DisabledEnum"=T6."Enabled" ("Disabled")) -> ()  [unwired: 2 in, 2 out]
                }
                frame True {
                  n382 = property on="Standby" class="Bool (strict)"("Val(Sgnl)"=TRUE ("Standby"), "DisabledEnum"=T6."Disabled" ("Disabled")) -> ()  [unwired: 2 in, 2 out]
                }
              }
              n383 = call "Resistivity_Calculation.vi"("Reading 1 (V)"=w1336, "Constant"="4PP constant", "Thickness (nm)"="Thickness (nm)", "Reading 2 (A)"=w1344) -> ("Resivtivity (Ohm*cm)"=w1328:dbl, "Current"=w1329:dbl, "Voltage"=w1330:dbl)
              "Resistivity (Ohm*cm)" <- w1328
              "Voltage (V)" <- w1330
              "Current (A)" <- w1329
              n384 = call "I3252_Edit_Temperature.vi"("Temp. String"=w1345) -> ("Temp. (°C)"=w1339:dbl)
              "(°C)" <- w1339
              n385 = Build Array (concatenate)(w1341, w1342) -> (w1338:dbl[])
              n386 = Build Array (concatenate)(w1340, w1339) -> (w1326:dbl[])
              n387 = Build Array (concatenate)(w1337, w1330) -> (w1335:dbl[])
              n388 = Build Array (concatenate)(w1334, w1329) -> (w1332:dbl[])
              n389 = Build Array (concatenate)(w1333, w1328) -> (w1331:dbl[])
              n390 = Build Array(w1330, w1329, w1328) -> (w1327:dbl[])
            }
            frame #5 {
              n391 = Bundle(w1362, w1381) -> (w1366:cluster{dbl[], dbl[]})  [unwired: 1 in]
              n392 = Bundle(w1362, w1380) -> (w1365:cluster{dbl[], dbl[]})  [unwired: 1 in]
              n393 = Bundle(w1362, w1379) -> (→"Pirani (VVP1 Scroll)":cluster{dbl[], dbl[]})  [unwired: 1 in]
              n394 = Bundle(w1362, w1378) -> (→"Pressure OpenPort":cluster{dbl[], dbl[]})  [unwired: 1 in]
              n395 = Bundle(w1362, w1385) -> (→"Thermocouple (Sample holder 1)":cluster{dbl[], dbl[]})  [unwired: 1 in]
              n396 = Build Array (concatenate)(w1360, w1359) -> (w1361:dbl[])
              n397 = Bundle(w1362, w1387) -> (→"Voltage":cluster{dbl[], dbl[]})  [unwired: 1 in]
              n398 = Bundle(w1362, w1388) -> (→"Current":cluster{dbl[], dbl[]})  [unwired: 1 in]
              n399 = Bundle(w1362, w1389) -> (→"Resistivity":cluster{dbl[], dbl[]})  [unwired: 1 in]
              n400 = Build Array(w1366, w1365) -> (→"TPG 1":cluster{dbl[], dbl[]}[])
              n401 = Bundle(w1362, w1361) -> (→"Pyrometer Temperature °C":cluster{dbl[], dbl[]})  [unwired: 1 in]
              n402 = Build Array (concatenate)(w1384, w1394, w1393, w1383, w1373, w1369, w1367) -> (w1401:dbl[])
              "appended array" <- w1401
            }
            frame #6 {
              n403 = Unbundle(w1412) -> ("COM out"=w1411:refnum<visa-resource-name>, "Cluster (Ausgang)"=w1410:errorcluster)
              n404 = Unbundle(w1409) -> ("COM out"=w1408:refnum<visa-resource-name>, "Cluster (Ausgang)"=w1407:errorcluster)
              n405 = call "Elapsed Time"("Time Target (s)"="Intervall (s)") -> ("Time has Elapsed"=w1405:bool)  [unwired: 11 in, 7 out]
              n406 = And(x="Write to File", y=w1405) -> (x .and. y?=w1403:bool)
              n407 = case shown="False" w1403 {
                tunnel: [w1434 w1440] -> w1426
                tunnel: "File Path" -> [w1434 w1438]
                tunnel: w1419 -> [_ w1436]
                frame False {
                  n408 = property on="Write to File" class="Bool (strict)"("Blinking"=FALSE) -> ()  [unwired: 2 in, 2 out]
                }
                frame True {
                  n409 = flat-sequence {
                    tunnel: [w1442] -> w1439
                    tunnel: w1438 -> [w1442]
                    tunnel: [w1441] -> w1437
                    tunnel: w1436 -> [w1441]
                    tunnel: [w1447] -> w1440
                    tunnel: w1439 -> [w1446]
                    tunnel: w1437 -> [w1445]
                    frame #0 {
                      n410 = property on="Write to File" class="Bool (strict)"("Blinking"=TRUE) -> ()  [unwired: 2 in, 2 out]
                    }
                    frame #1 {
                      n411 = call-poly <vilib>:"Write To Spreadsheet File.vi"("format (%.3f)"="%g", "append to file? (new file:F)"=TRUE ("transpose? (no:F)"), "1D data"=w1445, "file path (dialog if empty)"=w1446) -> ("new file path (Not A Path if cancelled)"=w1447:path)  [unwired: 4 in]
                    }
                  }
                }
              }
              n412 = Merge Errors(w1430, w1429, w1427, w1410, w1407) -> (w1428:errorcluster)
              n413 = call <vilib>:"Simple Error Handler.vi"("error in (no error)"=w1428) -> ("error?"=w1413:bool)  [unwired: 4 in, 4 out]
              n414 = local write "File Path"(w1426) -> ()
            }
            frame #7 {
              w1466 = u32 1000 ("y")
              n415 = Tick Count (ms)() -> (millisecond timer value=w1468:u32)
              n416 = Subtract(x=w1468, y=w1467) -> (x-y=w1469:u32)
              n417 = VISA Flush I/O Buffer(VISA resource name=w1460, error in (no error)=w1459) -> (VISA resource name out=w1457:refnum<visa-resource-name>, error out=w1458:errorcluster)  [unwired: 1 in]
              n418 = VISA Flush I/O Buffer(VISA resource name=w1453, error in (no error)=w1452) -> (VISA resource name out=w1456:refnum<visa-resource-name>, error out=w1455:errorcluster)  [unwired: 1 in]
              n419 = Divide(x=w1469, y=w1466) -> (x/y=→"loop time (s)":dbl)
              n420 = Subtract(x=u32 1, y=u32 1) -> (x-y=w1450:u32)
              n421 = Multiply(x=w1450, y=w1466) -> ()  [unwired: 1 out]
              n422 = Wait (ms)(milliseconds to wait=w1450) -> ()  [unwired: 1 out]
              n423 = Bundle("COM out"=w1457, "error out"=w1458, "COM out"=w1456, "error out"=w1455) -> (w1454:T12)  [unwired: 1 in]
            }
            frame #8 {
              n424 = Tick Count (ms)() -> (millisecond timer value=w1491:u32)
              n425 = Subtract(x=w1491, y=w1489) -> (x-y=w1490:u32)
              n426 = Divide(x=w1490, y=w1488) -> (x/y=→"data logger intervall (s)":dbl)
            }
          }
          n427 = Exclusive Or(1:"stop", 2:w185) -> (0:w186:bool)
        }
      }
      frame #4 {
        n428 = call "VC840_Close.vi"("error in (no error)"=w1511, "VISA resource name"=w1512) -> ("error out"=w1520:errorcluster)  [unwired: 9 in]
        n429 = call "VC840_Close.vi"("error in (no error)"=w1513, "VISA resource name"=w1514) -> ("error out"=w1518:errorcluster)  [unwired: 9 in]
        n430 = VISA Close(VISA resource name=w1516, error in (no error)=w1515) -> (error out=w1517:errorcluster)
        n431 = Unbundle(w1509) -> ("COM out"=w1508:refnum<visa-resource-name>, "error out"=w1507:errorcluster, "COM out"=w1505:refnum<visa-resource-name>, "error out"=w1506:errorcluster)
        n432 = VISA Close(VISA resource name=w1504) -> ()  [unwired: 1 in, 1 out]
        n433 = VISA Close(VISA resource name=w1508, error in (no error)=w1507) -> ()  [unwired: 1 out]
        n434 = VISA Close(VISA resource name=w1505, error in (no error)=w1506) -> ()  [unwired: 1 out]
        n435 = Merge Errors(w1517, w1518, w1520) -> (w1519:errorcluster)
        n436 = call <vilib>:"Simple Error Handler.vi"("error in (no error)"=w1519) -> ("error?"=w1510:bool)  [unwired: 1 in, 7 out]
        n437 = Stop(stop? (T)=w1510) -> ()
      }
    }
  }
